vi "App -- rpr -- view optimal subspace.vi"(10 "section index":i32=9) -> (0 "Array":dbl[][](array[numeric])=[[-0.6539993268930167, 0.3391236144564683, -0.09456432043806404, 0.0051367164973633896, 0.0020044244170662685, 0.011874272381953276, 0.06955451759566218, 0.007725271948397916, -0.004046329903722955, 0.012996231366623931, 0.02336389200775809, 0.024693616597254348, -0.043124477823421006, -0.017775933941850515, 0.04206965874272625, -0.11798708971321988, -0.08203489517148861, 0.015852951226723568, -0.06159173734444465, -0.0906144627663518, -0.048921335123773224, -0.025097551631409025, 0.03747376904568885, 0.026314885922756725, -0.08142107802798851, -0.04367395508948556, 0.025063497548666342, 0.037473769045688714, -0.09061446276635161, 0.07028982367908473, -0.037287084745676984, -0.03331452126771534, -0.0014293476377641413, -0.0291901136218296, 0.0446928180029198, 0.00290562753315699, 0.012066348733460198, 0.012562461680758148, -0.018476184956469036, 0.024652499530850507, -0.00011169769376606508, -0.043673955089485336, -0.034237925342999874, -0.041796842880443226, 0.03260096402459978, 0.013337833923163239, 0.028074032981141733, 0.02479303749859956, 0.04773146565334352, -0.0917979629943126, -0.08210132900667996, 0.07469329051450514, 0.04284862090477776, -0.048649980732486074, 0.05107537884702248, -0.045809372663442795, 0.12325677070152805, 0.05609768493174689, -0.002976243880241466, 0.055086131759920394, -0.010877679296898951, -0.029218379981849323, -0.010877679296900285, -0.048682509171851414, -0.08284375332862261, 0.11159983091108487, -0.02061373332521245, 0.07830420438142319, -0.05749858935992324, 0.030209847921128213, 0.033187881765827563, 0.0632454769770712, 0.011685909194376521, 0.014141087261257316, 0.09595339373441054, 0.034766252436734583, -0.06982174337419339, -0.0082770012246038, -0.02630887225081902, -0.09198148956369846, 0.011620057966691983, 0.012656148379396237, 0.02704444806042294, -0.055089665311336876, -0.010877679296900226, 0.11265218201672413, -0.027770881489970173, 0.014843280637345453, -0.023190740122303075, 0.057998283736627604, 0.025404299712243082, 0.05096886575937984, -0.011041283301146457, -0.0785294557445813, -0.1179870897132201, 0.01825031298729252, 0.004059220722186789, 0.009722439156744988, 0.06360381321170706, -0.03557589423855971, -0.03658151530191978, -0.059497458408195626, -0.019694269436186972, 0.07525056135337402, -0.04945967745638282, 0.02704444806042326, -0.023748803061154487, 0.054380122215328834, -0.07703437213244521, 0.08566875796505154, -0.020251331993503582, -0.023952284418691773, -0.02952998594490326, 0.04206965874272611, 0.015136067978359483, -0.07102312521130782, 0.04110574188038118, -0.047734799331777364, -0.009159302165546394, 0.05123083050100717, 0.16247491505060013, -0.03658151530191925, -0.04055517231337933, -0.06397759432387508, 0.05000696501163893, -0.02274052786555141, -0.036117801828781416, 0.06438911827431076, -0.06397759432387551, 0.07902148482902957, 0.07091125409732564, 0.05660232490132762, 0.003488096034465255, 0.06098287440769287, -0.07312812028096935, -0.03997679857564285, 0.06966129911814035, -0.01200735338094387, 0.0011683041305290498, -0.026973944618607863, 0.014809638246185298, 0.05660232490132767, -0.042969630453861575, -0.0008353715209700875, -0.009143131205386776, 0.04385368363874332, 0.03122354997581172, 0.023208866857712538, -0.011927566069049402, 0.011685909194375446, 0.01752271351681508, -0.016581982918802186, 0.014945230605948495, 0.00875427084575472, 0.03168710415197408, -0.01658087713761681, -0.006730271771716752, -0.006780822682695883, -0.04222734411828173, 0.0011683041305291441, 0.04477780338783405, 0.016848841839736322, 0.024236387665468876, 0.011563814441528143, 0.08814160730020291, 0.023632730480340702, -0.019314907742346392, 0.023208866857712732, 0.01770600216283244, 0.0034828877704507445, -0.030412875700733543, 0.02234017525324682, -0.04617557628949561, -0.06294948272567681, -0.009373798802334287, 0.026878262977207832, -0.052669278619909915, -0.0038344873940750553, 0.02897704740047952, 0.0040978082744671795, 0.04452617477957913, -0.11255781245377125, 0.04010898135209824, 0.0610473165358694, 0.02223933544743438, 0.02241750520192594, -0.007179708450721197, 0.0014508139903299858, 0.02491818912257842, -0.013717635945350942, 0.02357438582599947, 0.028669025739076148, 0.0536097823579598, -0.001068008136356144, 0.038631164135670075, -0.012463770264631075, 0.01336088595160985, 0.012451807078451239, -0.03804059074580767, 0.010373724593344768, 0.025629310861148537, -0.0053638644795241846, -0.012735855163042972, -0.05318586105391781], [-0.07067784298662909, -0.07185242549664024, -0.07144584854430172, -0.07119264899191084, -0.07332609474471392, -0.07070644115676238, -0.07084424275621311, -0.07075801362519098, -0.0712278012033401, -0.07029824202490799, -0.07206471962913785, -0.07100032939852118, -0.0702926266422602, -0.07144584854430172, -0.07079246391516397, -0.07139851601076179, -0.07310747635024652, -0.07331963305869194, -0.0728467622935989, -0.07102354972586497, -0.07108171016277974, -0.07138669909159649, -0.07391572105966812, -0.06813584333743469, -0.07145769792753225, -0.07104098139347476, -0.0699417731331728, -0.07391572105966812, -0.07102354972586497, -0.07357308458233423, -0.07010256843552296, -0.07051839030505405, -0.07022535585123252, -0.0715705929812706, -0.07089037299184926, -0.07132182152419132, -0.07098293054567185, -0.0719552788008493, -0.07094238772761886, -0.07107006552052214, -0.07104679508186065, -0.07104098139347476, -0.07106424555639645, -0.07101774229969898, -0.07116339918824471, -0.07589690867298654, -0.07205253207473776, -0.07197348041419911, -0.07248324864121716, -0.07161830511784921, -0.07200385061628492, -0.07207081599015004, -0.07193103385514005, -0.07170205620150355, -0.07239641439185673, -0.07265797313696364, -0.0727773475602805, -0.07229760149533275, -0.0728657324255394, -0.07186450045604705, -0.0718886706764948, -0.07125126788349785, -0.0718886706764948, -0.07137488864390973, -0.07145177242208574, -0.07318438297654763, -0.07192497687519935, -0.07072361827988241, -0.0714399262932863, -0.07467961351717668, -0.07194315292089142, -0.07124539881911628, -0.07097713404598982, -0.07123953135154178, -0.07230376405486523, -0.0738097134634255, -0.07213187457266167, -0.07481075543571364, -0.07131004654331616, -0.07114002787526968, -0.0698150928635247, -0.07075227725677384, -0.07086153003324067, -0.07168408213995159, -0.0718886706764948, -0.07086729553974122, -0.07085576606770128, -0.07181624113087454, -0.07060936171097355, -0.07080970971931133, -0.0714340056681463, -0.07070071848804443, -0.06955851567785098, -0.07132771142643664, -0.07139851601076179, -0.07117509434956008, -0.07078671837711563, -0.07337785805054228, -0.07087883117892353, -0.07055245962799597, -0.07046172743237006, -0.07099452822109902, -0.07008031836706796, -0.07092503553925854, -0.07252679723197354, -0.07086153003324067, -0.06924603934869149, -0.0709192545777074, -0.07057520244785964, -0.07069499733747715, -0.0699086542985036, -0.06971646825442701, -0.06993072786945531, -0.07079246391516397, -0.07002479342152154, -0.07009144053179982, -0.07017504010775154, -0.07010813454135774, -0.06976572418052975, -0.0699915469448388, -0.07082696932562439, -0.07046172743237006, -0.07047304810293813, -0.07013598663994308, -0.06967823571596993, -0.06965641894431973, -0.06949349288405872, -0.06971100231169412, -0.07013598663994308, -0.06959653637490698, -0.06935327913673697, -0.06994729788712568, -0.0694017115694283, -0.06943406039089926, -0.06992520735824197, -0.06889062268192965, -0.06933178847533021, -0.069732874399712, -0.0683246384498748, -0.06848410063974669, -0.06874380846205878, -0.06994729788712568, -0.06895385031657847, -0.0696509681981926, -0.0690384432249917, -0.0693855553367308, -0.06952056189343293, -0.06818670627831608, -0.0683502785396113, -0.07097713404598982, -0.06816125981290112, -0.06852027200046291, -0.06892748293716348, -0.06768339575801093, -0.06809523917964166, -0.06912336925918049, -0.0663429299804043, -0.06828367760767108, -0.06710905713668458, -0.0683246384498748, -0.06814092423672478, -0.06639910334041323, -0.06645072443922147, -0.06837081258252144, -0.06774816568082924, -0.06748531512839379, -0.06714299243391042, -0.06818670627831608, -0.06797892627732868, -0.06705100628888166, -0.06637099837083553, -0.06515159427912529, -0.06755938232290597, -0.06754454851954433, -0.06711874748820106, -0.0682172817233295, -0.06716726466712766, -0.0677981214060557, -0.06712844219591076, -0.06614746752208296, -0.06816634670452446, -0.0700469862477013, -0.06684426460786311, -0.06985356901456403, -0.06499292371464982, -0.06696903415934995, -0.06927279934336097, -0.06700274966338278, -0.06596294552418623, -0.06483541204473581, -0.06636163818104576, -0.06625428698663569, -0.06589415478982338, -0.0669642219587416, -0.06759898908690724, -0.066582683888146, -0.06609194495907281, -0.06578910000841474, -0.06506770602475595, -0.06488778821361832, -0.06546799157784904, -0.06563020955326251, -0.06601813653815264, -0.06577543486257549]], 1 "Array of clasters":cluster{"temperature points OUT":dbl[], dbl[]}[](array[cluster])=[{"temperature points OUT"=[55.393, 55.473, 55.549, 55.623, 55.697, 55.77, 55.847, 55.926, 56.007, 56.087, 56.169, 56.251, 56.332, 56.409, 56.489, 56.565, 56.645, 56.724, 56.8, 56.877, 56.955, 57.034, 57.114, 57.191, 57.269, 57.348, 57.425, 57.505, 57.583, 57.656, 57.736, 57.815, 57.896, 57.974, 58.055, 58.137, 58.217, 58.295, 58.373, 58.45, 58.526, 58.605, 58.679, 58.759, 58.836, 58.913, 58.989, 59.071, 59.148, 59.226, 59.302, 59.381, 59.459, 59.539, 59.616, 59.694, 59.77, 59.846, 59.925, 59.998, 60.076, 60.154, 60.23, 60.308, 60.384, 60.462, 60.54, 60.618, 60.693, 60.77, 60.849, 60.928, 61.004, 61.082, 61.16, 61.239, 61.315, 61.391, 61.468, 61.544, 61.626, 61.703, 61.781, 61.86, 61.93, 62.009, 62.083, 62.162, 62.238, 62.312, 62.389, 62.466, 62.541, 62.618, 62.697, 62.774, 62.854, 63.013, 63.088, 63.165, 63.241, 63.317, 63.394, 63.472, 63.549, 63.628, 63.705, 63.782, 63.861, 63.937, 64.014, 64.089, 64.162, 64.239, 64.316, 64.393, 64.47, 64.547, 64.62, 64.696, 64.817, 64.892, 64.971, 65.046, 65.123, 65.2, 65.275, 65.35, 65.429, 65.507, 65.582, 65.655, 65.733, 65.81, 65.887, 65.965, 66.042, 66.193, 66.27, 66.345, 66.423, 66.5, 66.574, 66.651, 66.728, 66.802, 66.881, 66.956, 67.032, 67.108, 67.187, 67.258, 67.335, 67.411, 67.487, 67.563, 67.639, 67.717, 67.792, 67.869, 67.941, 68.018, 68.097, 68.174, 68.251, 68.349, 68.484, 68.558, 68.632, 68.708, 68.787, 68.864, 69.014, 69.092, 69.169, 69.246, 69.323, 69.397, 69.472, 69.546, 69.621, 69.696, 69.771, 69.845, 69.924, 69.997, 70.071, 70.149, 70.225, 70.301, 70.381, 70.457, 70.533, 70.609, 70.682, 70.76, 70.84, 70.915, 70.993, 71.145, 71.222, 71.3, 71.374, 71.452], [-1.4233131947990045, -1.44696698379756, -1.4387793210660562, -1.4336803784751888, -1.4766437933452072, -1.4238891058791603, -1.4266641599339325, -1.4249276742861876, -1.4343882750979413, -1.4156687756324693, -1.4512421714262957, -1.429807438904274, -1.4155556928348239, -1.4387793210660562, -1.4256214355869177, -1.4378261366353517, -1.472241247479028, -1.476513667656772, -1.4669909775045147, -1.430275050773841, -1.4314462879505574, -1.4375881670502726, -1.4885177113739985, -1.3721223054200284, -1.4390179444137645, -1.4306260903849541, -1.4084901910053458, -1.4885177113739985, -1.430275050773841, -1.4816176844546562, -1.411728293157671, -1.4201021303968961, -1.414200990986999, -1.4412914294668342, -1.4275931324419442, -1.4362816600343222, -1.4294570601181025, -1.449038247701824, -1.4286406072461604, -1.431211787684653, -1.43074316667139, -1.4306260903849541, -1.4310945850171213, -1.4301581005962385, -1.4330913447731966, -1.5284149458148104, -1.4509967379742121, -1.4494047925106721, -1.4596705252091262, -1.4422522583585318, -1.4500163888403113, -1.4513649401852484, -1.448550002027125, -1.4439388409904674, -1.4579218536643743, -1.4631891340084586, -1.465593100862123, -1.4559319556497243, -1.4673729987711088, -1.447210149807218, -1.447696890661646, -1.4348608480302105, -1.447696890661646, -1.4373503277880832, -1.438898616350944, -1.4737899961583356, -1.4484280263257463, -1.4242350194632807, -1.4386600585410987, -1.5039010078674286, -1.4487940562520938, -1.4347426565797863, -1.429340329978466, -1.4346244972859263, -1.4560560575170935, -1.486382926212125, -1.4525945403325102, -1.5065419490048115, -1.4360445350041873, -1.4326206923490212, -1.4059390987295817, -1.424812155072339, -1.427012291801795, -1.4435768786287146, -1.447696890661646, -1.4271283977995197, -1.4268962168360089, -1.4462383016099956, -1.4219341161639085, -1.4259687322722812, -1.438540828758084, -1.423773862550395, -1.4007721372262036, -1.436400271118469, -1.4378261366353517, -1.4333268623938835, -1.4255057317146724, -1.4776862048433326, -1.4273607029571869, -1.420788219768501, -1.4189610512278328, -1.4296906145641202, -1.4112802203999435, -1.4282911681913124, -1.4605475084505393, -1.427012291801795, -1.394479476562531, -1.428174750959171, -1.4212462155735655, -1.4236586497942072, -1.407823242604133, -1.4039529924545608, -1.4082677610481644, -1.4256214355869177, -1.4101620568525401, -1.41150419899279, -1.413187730556624, -1.411840383616908, -1.4049449102406961, -1.4094925379914167, -1.426316306906202, -1.4189610512278328, -1.4191890273390537, -1.412401270278755, -1.4031830640844094, -1.4027437170748582, -1.399462705635531, -1.4038429190838275, -1.412401270278755, -1.4015377995258496, -1.3966390756516194, -1.4086014487187513, -1.3976144098948948, -1.3982658517398951, -1.4081565887752154, -1.3873220816834984, -1.396206295863037, -1.4042833800565757, -1.3759242688543174, -1.3791355247348789, -1.384365531122584, -1.4086014487187513, -1.3885953622884066, -1.4026339497339722, -1.3902988976206005, -1.3972890550424426, -1.400007822415902, -1.3731465853332743, -1.376440609994563, -1.429340329978466, -1.3726341434072673, -1.3798639450262424, -1.3880643749598776, -1.3630108981877709, -1.3713046172859766, -1.392009141452825, -1.3360165453917334, -1.3750993977955097, -1.3514448443373293, -1.3759242688543174, -1.372224624770697, -1.3371477667352039, -1.3381873144627388, -1.3768541253620603, -1.3643152374527774, -1.3590219426416679, -1.3521282346937675, -1.3731465853332743, -1.3689623034632596, -1.3502758140704776, -1.3365817877473203, -1.3120253799654444, -1.360513510731414, -1.3602147870131798, -1.3516399890190685, -1.3737623148530995, -1.3526170298853801, -1.3653212478213177, -1.351835221425999, -1.3320803146826385, -1.372736583431779, -1.410608976863067, -1.3461124419290225, -1.4067139329795428, -1.308830065868396, -1.3486250560869568, -1.3950183703925685, -1.3493040202393891, -1.3283644033978703, -1.3056580896358188, -1.3363932918754797, -1.3342314492806202, -1.3269790928711038, -1.3485281478009576, -1.3613111133098765, -1.3408447190593702, -1.3309621991148441, -1.324863495532006, -1.3103360349842297, -1.3067128429943444, -1.3183970012691315, -1.32166375326782, -1.32947584221792, -1.3245883062851367]}], 11 "9w folder path":path=path "E:/data/Ultrasound/Experiment/ProbeTest/Probe10/YBCO_5/sweep5/9w")   [LabVIEW 2014]
uses:
  link -- rusout - tetragonal.ctl
  cursor winow.ctl
  query.ctl
  cursor window action.ctl
  <vilib>/Analysis/baseanly.llb/Real A x B.vi
  <vilib>/Utility/file.llb/Write To Spreadsheet File (DBL).vi
  <vilib>/Analysis/Matrix/Numeric/Conversions/Array To Matrix - RA2.vi
  <vilib>/Analysis/Matrix/Numeric/Conversions/Matrix To Array - RM.vi
  <vilib>/Analysis/Matrix/NI_Matrix.lvlib
  <vilib>/Analysis/NI_AALBase.lvlib
panel:
  in  "Tab Control 2":enum32{"Page 1", "Page 2"}(tab)
  out "Plot:   what vs temp 2":cluster{dbl[], dbl[]}[](graph)=[{[60.693, 60.77, 60.849, 60.928, 61.004, 61.082, 61.16, 61.239, 61.315, 61.391, 61.468, 61.544, 61.626, 61.703, 61.781, 61.86, 61.93, 62.009, 62.083, 62.162, 62.238, 62.312, 62.389, 62.466, 62.541, 62.618, 62.697, 62.774, 62.854, 62.932, 63.013, 63.088, 63.165, 63.241, 63.317, 63.394, 63.472, 63.549], [-0.0004933279279327732, -0.0004959461002016808, -0.0004987375917983193, -0.0005013767724705882, -0.0005039476758319328, -0.0005070674237310925, -0.0005096724657478992, -0.0005120936842352941, -0.0005132649027226891, -0.0005130075497815126, -0.0005117076548235294, -0.0005095096506218488, -0.0005068126968403361, -0.0005043625917983194, -0.0005024770875966387, -0.0005009854909579832, -0.0005000269825546219, -0.0004992365413781513, -0.0004986719405378152, -0.0004978683691092438, -0.0004972249867563025, -0.000496810070789916, -0.0004963557640672269, -0.000495951352302521, -0.0004956414783529412, -0.0004949140623865546, -0.0004947512472605043, -0.0004943310791932774, -0.0004938058691092437, -0.0004934907430588235, -0.000493107339697479, -0.0004928132220504202, -0.0004925007220504202, -0.0004922880119663866, -0.0004920805539831933, -0.0004917207850756302, -0.0004911640623865547, -0.000490856814487395]}, {[60.693, 60.77, 60.849, 60.928, 61.004, 61.082, 61.16], [-0.0004933414395167107, -0.0004959475211230401, -0.0004986595074246494, -0.0005014110372937718, -0.0005040962098828075, -0.0005068917751889707, -0.0005097284672831535]}, {[61.391, 61.468, 61.544, 61.626, 61.703, 61.781], [-0.0005134949407613455, -0.0005112990207351107, -0.00050914039550645, -0.0005068210704880685, -0.0005046522940388857, -0.0005024643077469364]}]
  out "best fit parameters right":dbl[](array[numeric])=[0.000561899976493353, -0.040468997251097254, -37.63175425304014]
  out "best fit parameters left":dbl[](array[numeric])=[-0.0001212473626486651, -0.0041194510604749875, -10.603993376591303]
  in  "gap":dbl=1.0
  out "residue right":dbl=1.0417365940205689e-13
  out "residue left":dbl=9.072396572402669e-15
  out "x-y":dbl[](array[numeric])=[-3.1383182947303852e-06, -3.7664734781920825e-06, 1.2053722232650138e-06]
  out "Plot:   LandauKhalat":cluster{"Array":dbl[], dbl[]}[](graph)
  out "Plot:   optimal subspace derivative":cluster{dbl[], dbl[]}[](graph)=[{[55.393, 55.473, 55.549, 55.623, 55.697, 55.77, 55.847, 55.926, 56.007, 56.087, 56.169, 56.251, 56.332, 56.409, 56.489, 56.565, 56.645, 56.724, 56.8, 56.877, 56.955, 57.034, 57.114, 57.191, 57.269, 57.348, 57.425, 57.505, 57.583, 57.656, 57.736, 57.815, 57.896, 57.974, 58.055, 58.137, 58.217, 58.295, 58.373, 58.45, 58.526, 58.605, 58.679, 58.759, 58.836, 58.913, 58.989, 59.071, 59.148, 59.226, 59.302, 59.381, 59.459, 59.539, 59.616, 59.694, 59.77, 59.846, 59.925, 59.998, 60.076, 60.154, 60.23, 60.308, 60.384, 60.462, 60.54, 60.618, 60.693, 60.77, 60.849, 60.928, 61.004, 61.082, 61.16, 61.239, 61.315, 61.391, 61.468, 61.544, 61.626, 61.703, 61.781, 61.86, 61.93, 62.009, 62.083, 62.162, 62.238, 62.312, 62.389, 62.466, 62.541, 62.618, 62.697, 62.774, 62.854, 63.013, 63.088, 63.165, 63.241, 63.317, 63.394, 63.472, 63.549, 63.628, 63.705, 63.782, 63.861, 63.937, 64.014, 64.089, 64.162, 64.239, 64.316, 64.393, 64.47, 64.547, 64.62, 64.696, 64.817, 64.892, 64.971, 65.046, 65.123, 65.2, 65.275, 65.35, 65.429, 65.507, 65.582, 65.655, 65.733, 65.81, 65.887, 65.965, 66.042, 66.193, 66.27, 66.345, 66.423, 66.5, 66.574, 66.651, 66.728, 66.802, 66.881, 66.956, 67.032, 67.108, 67.187, 67.258, 67.335, 67.411, 67.487, 67.563, 67.639, 67.717, 67.792, 67.869, 67.941, 68.018, 68.097, 68.174, 68.251, 68.349, 68.484, 68.558, 68.632, 68.708, 68.787, 68.864, 69.014, 69.092, 69.169, 69.246, 69.323, 69.397, 69.472, 69.546, 69.621, 69.696, 69.771, 69.845, 69.924, 69.997, 70.071, 70.149, 70.225, 70.301, 70.381, 70.457, 70.533, 70.609, 70.682, 70.76, 70.84, 70.915, 70.993, 71.145, 71.222, 71.3, 71.374, 71.452], [0.0, 12.414036766868827, -5.706420195980651, 1.3473113099382437, -0.04232827135536354, 0.13520339677927334, 0.7490940936845489, -0.7826486790792884, -0.1453284179274254, 0.21303201587932172, 0.12643488586749957, 0.016216153530442028, -0.8372604249465776, 0.3292018685918323, 0.7480699085572255, -2.10600984810454, 0.4494024317716105, 1.2390866632686104, -1.0190090601469433, -0.3769185119727942, 0.5345272774689844, 0.30156687965017737, 0.7821415084637401, -0.14492056003806963, -1.3812303070609098, 0.47781168276585634, 0.8926941901058899, 0.15512839371276918, -1.6421568181031685, 2.204168307471719, -1.3447113553095502, 0.05028561364508367, 0.3936441188882715, -0.35590725620598634, 0.912134958330205, -0.5095998837775906, 0.11450901500379254, 0.00636042240125553, -0.39793136714395944, 0.560112785549566, -0.3258447003239001, -0.5514209796926942, 0.12751391549303787, -0.09448646921804392, 0.9662052844811007, -0.250170520797883, 0.1938973560260315, -0.04001214003100173, 0.2979016643473037, -1.7888388288161992, 0.12758728931095492, 1.984742019255492, -0.4082649949964895, -1.1437325204658224, 1.2951345399936482, -1.2421121988520718, 2.2245545179601276, -0.8836721811814078, -0.7477712507846568, 0.7953750087693362, -0.8456898853438056, -0.2351371882685856, 0.24132500901250825, -0.4846773060890987, -0.44949005469435477, 2.4928664646115397, -1.6950456953372353, 1.2681786885465627, -1.8107039165513887, 1.1390706140395512, 0.03769663094556448, 0.3804758887499164, -0.6784153655617674, 0.031476641883085923, 1.0488757240148407, -0.7745207759199427, -1.376157839617464, 0.8097992388103838, -0.23418014319758418, -0.8641133856958572, 1.2634335064681648, 0.013455719645508873, 0.18446538052599318, -1.0396723211615084, 0.6315998002062353, 1.5636691305521946, -1.8976089663067295, 0.5394197737634847, -0.5004476415743193, 1.0971489710666593, -0.42329849382314655, 0.33200735126152414, -0.8268019874737309, -0.8764697719926001, -0.49946372112200615, 1.7693169181885176, -0.17738865331382542, 0.03561772600351092, 0.7184183207328004, -1.2880481487047937, -0.013231856096842968, -0.301525567187838, 0.5169245321040208, 1.217241420378941, -1.6196134910358415, 0.9684066521114617, -0.6596526119685577, 1.0146613672270801, -1.6634746119971267, 2.1408306591775745, -1.3755855838773716, -0.04934603233584067, -0.07640687022206732, 0.92986551542378, -0.34978689304373073, -1.1189505609047967, 1.4562190531388528, -1.1537732624955928, 0.528431468030507, 0.7946070087705105, 0.9193725995834501, -2.654085738033491, -0.05029945584126193, -0.31229896013993147, 1.4803189524093079, -0.9447726347687281, -0.17836365284306002, 1.3400922680414322, -1.624895096179414, 1.8333215276012778, -0.10813640975606878, -0.1960127287122815, -0.6809516521392353, 0.7466854334185582, -1.741701229722927, 0.42501694494006725, 1.4238713986205946, -0.540852003305207, 0.17111243521393807, -0.3752299833218113, 0.5356869598050202, 0.5427621643525111, -1.3455669642593493, 0.5471981679596426, -0.10789298291450498, 0.7161731735692067, -0.15987510965737514, -0.1068624415746517, -0.4623214858784867, 0.3107036218871379, 0.07388359901822927, -0.48034783712138385, 0.4094443314902782, -0.08145999684464678, 0.30174780666080725, -0.6351050169682376, 0.12961322849869622, -0.0006480886022965323, -0.47262028580779336, 0.5635798473871676, 0.6056874896847674, -0.3627137863389401, 0.09351323830041974, -0.16457887303816485, 0.9945167903724231, -0.6582538451006417, -0.3181306535014073, 0.5746456027034064, -0.07436303641730319, -0.18714624200503854, -0.4290602971035566, 0.685104557843917, -0.45677167695164217, -0.21505008251513544, 0.6957881029005687, 0.4708059971369218, -1.0330849558067483, 0.6599296111598211, 0.43748713059412736, -0.33620593413524613, 0.5390448867349077, -2.094453163111259, 2.0355572507448496, 0.2829504754563744, -0.4912402669421674, 0.002440681568377736, -0.39996234665740416, 0.1106477236032161, 0.30878125174013776, -0.5083661193148091, 0.46615027214189003, 0.06703473569838315, 0.32816785024843625, -0.7194446117673775, 0.5438242776989334, -0.6550632615422975, 0.3228082027030184, -0.012121051642114345, -0.6473384336444384, 0.3185152324944218, 0.1981244969844692, -0.39734840180348135, -0.09962149572322947, -0.5185898191137603]}, ...(2 in all)]
  out "standard error":string
  out "standard output":string
  out "string":string
  out "name":string
  out "Numeric":i32=1
  out "common  freq points":dbl[][](array[numeric])=[[-1.4233131947990045, -1.44696698379756, -1.4387793210660562, -1.4336803784751888, -1.4766437933452072, -1.4238891058791603, -1.4266641599339325, -1.4249276742861876, -1.4343882750979413, -1.4156687756324693, -1.4512421714262957, -1.429807438904274, -1.4155556928348239, -1.4387793210660562, -1.4256214355869177, -1.4378261366353517, -1.472241247479028, -1.476513667656772, -1.4669909775045147, -1.430275050773841, -1.4314462879505574, -1.4375881670502726, -1.4885177113739985, -1.3721223054200284, -1.4390179444137645, -1.4306260903849541, -1.4084901910053458, -1.4885177113739985, -1.430275050773841, -1.4816176844546562, -1.411728293157671, -1.4201021303968961, -1.414200990986999, -1.4412914294668342, -1.4275931324419442, -1.4362816600343222, -1.4294570601181025, -1.449038247701824, -1.4286406072461604, -1.431211787684653, -1.43074316667139, -1.4306260903849541, -1.4310945850171213, -1.4301581005962385, -1.4330913447731966, -1.5284149458148104, -1.4509967379742121, -1.4494047925106721, -1.4596705252091262, -1.4422522583585318, -1.4500163888403113, -1.4513649401852484, -1.448550002027125, -1.4439388409904674, -1.4579218536643743, -1.4631891340084586, -1.465593100862123, -1.4559319556497243, -1.4673729987711088, -1.447210149807218, -1.447696890661646, -1.4348608480302105, -1.447696890661646, -1.4373503277880832, -1.438898616350944, -1.4737899961583356, -1.4484280263257463, -1.4242350194632807, -1.4386600585410987, -1.5039010078674286, -1.4487940562520938, -1.4347426565797863, -1.429340329978466, -1.4346244972859263, -1.4560560575170935, -1.486382926212125, -1.4525945403325102, -1.5065419490048115, -1.4360445350041873, -1.4326206923490212, -1.4059390987295817, -1.424812155072339, -1.427012291801795, -1.4435768786287146, -1.447696890661646, -1.4271283977995197, -1.4268962168360089, -1.4462383016099956, -1.4219341161639085, -1.4259687322722812, -1.438540828758084, -1.423773862550395, -1.4007721372262036, -1.436400271118469, -1.4378261366353517, -1.4333268623938835, -1.4255057317146724, -1.4776862048433326, -1.4273607029571869, -1.420788219768501, -1.4189610512278328, -1.4296906145641202, -1.4112802203999435, -1.4282911681913124, -1.4605475084505393, -1.427012291801795, -1.394479476562531, -1.428174750959171, -1.4212462155735655, -1.4236586497942072, -1.407823242604133, -1.4039529924545608, -1.4082677610481644, -1.4256214355869177, -1.4101620568525401, -1.41150419899279, -1.413187730556624, -1.411840383616908, -1.4049449102406961, -1.4094925379914167, -1.426316306906202, -1.4189610512278328, -1.4191890273390537, -1.412401270278755, -1.4031830640844094, -1.4027437170748582, -1.399462705635531, -1.4038429190838275, -1.412401270278755, -1.4015377995258496, -1.3966390756516194, -1.4086014487187513, -1.3976144098948948, -1.3982658517398951, -1.4081565887752154, -1.3873220816834984, -1.396206295863037, -1.4042833800565757, -1.3759242688543174, -1.3791355247348789, -1.384365531122584, -1.4086014487187513, -1.3885953622884066, -1.4026339497339722, -1.3902988976206005, -1.3972890550424426, -1.400007822415902, -1.3731465853332743, -1.376440609994563, -1.429340329978466, -1.3726341434072673, -1.3798639450262424, -1.3880643749598776, -1.3630108981877709, -1.3713046172859766, -1.392009141452825, -1.3360165453917334, -1.3750993977955097, -1.3514448443373293, -1.3759242688543174, -1.372224624770697, -1.3371477667352039, -1.3381873144627388, -1.3768541253620603, -1.3643152374527774, -1.3590219426416679, -1.3521282346937675, -1.3731465853332743, -1.3689623034632596, -1.3502758140704776, -1.3365817877473203, -1.3120253799654444, -1.360513510731414, -1.3602147870131798, -1.3516399890190685, -1.3737623148530995, -1.3526170298853801, -1.3653212478213177, -1.351835221425999, -1.3320803146826385, -1.372736583431779, -1.410608976863067, -1.3461124419290225, -1.4067139329795428, -1.308830065868396, -1.3486250560869568, -1.3950183703925685, -1.3493040202393891, -1.3283644033978703, -1.3056580896358188, -1.3363932918754797, -1.3342314492806202, -1.3269790928711038, -1.3485281478009576, -1.3613111133098765, -1.3408447190593702, -1.3309621991148441, -1.324863495532006, -1.3103360349842297, -1.3067128429943444, -1.3183970012691315, -1.32166375326782, -1.32947584221792, -1.3245883062851367]]
  in  "Tab Control":T1(tab)
  in  "temperature mapping":bool
  in  "dump optimal vectors":bool
  in  "misc controls":T2[](array[typedef])=[{"Boolean"=FALSE, "String"="calc el consts"}, {"Boolean"=FALSE, "String"="read rusout file"}, {"Boolean"=FALSE, "String"="export plot "}, {"Boolean"=FALSE, "String"="critical"}]
  in  "buttons 4":bool[](array[boolean])=[FALSE, FALSE, TRUE, TRUE, TRUE, FALSE, FALSE, TRUE, FALSE, FALSE, TRUE, TRUE, FALSE, FALSE, FALSE, TRUE]
  in  "active":bool[](array[boolean])=[FALSE, TRUE, FALSE, FALSE]
  in  "buttons 3":bool[](array[boolean])=[FALSE, FALSE, FALSE, TRUE, FALSE, FALSE, FALSE, FALSE, FALSE, FALSE, FALSE, FALSE, FALSE, FALSE, FALSE, FALSE, FALSE, FALSE, FALSE, FALSE, FALSE, FALSE]
  in  "buttons 2":bool[](array[boolean])=[TRUE, TRUE, TRUE, TRUE, TRUE, TRUE, FALSE, TRUE, TRUE, FALSE, TRUE, TRUE, TRUE, TRUE, TRUE, TRUE, TRUE, TRUE, FALSE, FALSE, FALSE, FALSE]
  in  "show plot pallettes":bool
  out "Plot:   what vs temp":cluster{dbl[], dbl[]}[](graph)=[{[55.393, 55.473, 55.549, 55.623, 55.697, 55.77, 55.847, 55.926, 56.007, 56.087, 56.169, 56.251, 56.332, 56.409, 56.489, 56.565, 56.645, 56.724, 56.8, 56.877, 56.955, 57.034, 57.114, 57.191, 57.269, 57.348, 57.425, 57.505, 57.583, 57.656, 57.736, 57.815, 57.896, 57.974, 58.055, 58.137, 58.217, 58.295, 58.373, 58.45, 58.526, 58.605, 58.679, 58.759, 58.836, 58.913, 58.989, 59.071, 59.148, 59.226, 59.302, 59.381, 59.459, 59.539, 59.616, 59.694, 59.77, 59.846, 59.925, 59.998, 60.076, 60.154, 60.23, 60.308, 60.384, 60.462, 60.54, 60.618, 60.693, 60.77, 60.849, 60.928, 61.004, 61.082, 61.16, 61.239, 61.315, 61.391, 61.468, 61.544, 61.626, 61.703, 61.781, 61.86, 61.93, 62.009, 62.083, 62.162, 62.238, 62.312, 62.389, 62.466, 62.541, 62.618, 62.697, 62.774, 62.854, 63.013, 63.088, 63.165, 63.241, 63.317, 63.394, 63.472, 63.549, 63.628, 63.705, 63.782, 63.861, 63.937, 64.014, 64.089, 64.162, 64.239, 64.316, 64.393, 64.47, 64.547, 64.62, 64.696, 64.817, 64.892, 64.971, 65.046, 65.123, 65.2, 65.275, 65.35, 65.429, 65.507, 65.582, 65.655, 65.733, 65.81, 65.887, 65.965, 66.042, 66.193, 66.27, 66.345, 66.423, 66.5, 66.574, 66.651, 66.728, 66.802, 66.881, 66.956, 67.032, 67.108, 67.187, 67.258, 67.335, 67.411, 67.487, 67.563, 67.639, 67.717, 67.792, 67.869, 67.941, 68.018, 68.097, 68.174, 68.251, 68.349, 68.484, 68.558, 68.632, 68.708, 68.787, 68.864, 69.014, 69.092, 69.169, 69.246, 69.323, 69.397, 69.472, 69.546, 69.621, 69.696, 69.771, 69.845, 69.924, 69.997, 70.071, 70.149, 70.225, 70.301, 70.381, 70.457, 70.533, 70.609, 70.682, 70.76, 70.84, 70.915, 70.993, 71.145, 71.222, 71.3, 71.374, 71.452], [-1.4233131928950045, -1.44696698189356, -1.4387793191620561, -1.4336803765711887, -1.4766437914412072, -1.4238891039751602, -1.4266641580299324, -1.4249276723821875, -1.4343882731939412, -1.4156687737284692, -1.4512421695222957, -1.429807437000274, -1.4155556909308238, -1.4387793191620561, -1.4256214336829176, -1.4378261347313517, -1.472241245575028, -1.476513665752772, -1.4669909756005146, -1.430275048869841, -1.4314462860465573, -1.4375881651462725, -1.4885177094699984, -1.3721223035160284, -1.4390179425097644, -1.430626088480954, -1.4084901891013457, -1.4885177094699984, -1.430275048869841, -1.4816176825506562, -1.4117282912536708, -1.420102128492896, -1.414200989082999, -1.4412914275628341, -1.4275931305379441, -1.4362816581303222, -1.4294570582141024, -1.449038245797824, -1.4286406053421603, -1.431211785780653, -1.4307431647673898, -1.430626088480954, -1.4310945831131212, -1.4301580986922384, -1.4330913428691965, -1.5284149439108103, -1.450996736070212, -1.449404790606672, -1.4596705233051261, -1.4422522564545317, -1.4500163869363112, -1.4513649382812484, -1.4485500001231248, -1.4439388390864674, -1.4579218517603743, -1.4631891321044586, -1.465593098958123, -1.4559319537457243, -1.4673729968671088, -1.447210147903218, -1.447696888757646, -1.4348608461262105, -1.447696888757646, -1.4373503258840832, -1.438898614446944, -1.4737899942543355, -1.4484280244217462, -1.4242350175592806, -1.4386600566370986, -1.5039010059634286, -1.4487940543480937, -1.4347426546757862, -1.4293403280744659, -1.4346244953819263, -1.4560560556130935, -1.486382924308125, -1.4525945384285102, -1.5065419471008115, -1.4360445331001872, -1.4326206904450212, -1.4059390968255816, -1.4248121531683389, -1.4270122898977948, -1.4435768767247146, -1.447696888757646, -1.4271283958955197, -1.4268962149320088, -1.4462382997059955, -1.4219341142599085, -1.425968730368281, -1.438540826854084, -1.423773860646395, -1.4007721353222036, -1.4364002692144688, -1.4378261347313517, -1.4333268604898834, -1.4255057298106724, -1.4776862029393325, -1.4273607010531868, -1.4207882178645008, -1.4189610493238327, -1.42969061266012, -1.4112802184959434, -1.4282911662873123, -1.4605475065465392, -1.4270122898977948, -1.394479474658531, -1.4281747490551708, -1.4212462136695654, -1.4236586478902071, -1.407823240700133, -1.4039529905505608, -1.4082677591441644, -1.4256214336829176, -1.41016205494854, -1.4115041970887898, -1.413187728652624, -1.411840381712908, -1.404944908336696, -1.4094925360874166, -1.4263163050022019, -1.4189610493238327, -1.4191890254350537, -1.4124012683747549, -1.4031830621804093, -1.4027437151708582, -1.399462703731531, -1.4038429171798275, -1.4124012683747549, -1.4015377976218495, -1.3966390737476193, -1.4086014468147512, -1.3976144079908948, -1.398265849835895, -1.4081565868712154, -1.3873220797794983, -1.396206293959037, -1.4042833781525756, -1.3759242669503173, -1.3791355228308788, -1.384365529218584, -1.4086014468147512, -1.3885953603844066, -1.402633947829972, -1.3902988957166005, -1.3972890531384425, -1.400007820511902, -1.3731465834292742, -1.376440608090563, -1.4293403280744659, -1.3726341415032672, -1.3798639431222424, -1.3880643730558775, -1.3630108962837708, -1.3713046153819766, -1.392009139548825, -1.3360165434877334, -1.3750993958915096, -1.3514448424333292, -1.3759242669503173, -1.372224622866697, -1.3371477648312038, -1.3381873125587387, -1.3768541234580602, -1.3643152355487773, -1.3590219407376678, -1.3521282327897675, -1.3731465834292742, -1.3689623015592596, -1.3502758121664775, -1.3365817858433202, -1.3120253780614444, -1.3605135088274138, -1.3602147851091797, -1.3516399871150684, -1.3737623129490995, -1.35261702798138, -1.3653212459173176, -1.351835219521999, -1.3320803127786385, -1.372736581527779, -1.410608974959067, -1.3461124400250224, -1.4067139310755428, -1.308830063964396, -1.3486250541829568, -1.3950183684885684, -1.349304018335389, -1.3283644014938703, -1.3056580877318187, -1.3363932899714797, -1.3342314473766201, -1.3269790909671038, -1.3485281458969576, -1.3613111114058765, -1.3408447171553701, -1.330962197210844, -1.324863493628006, -1.3103360330802296, -1.3067128410903444, -1.3183969993651314, -1.3216637513638199, -1.32947584031392, -1.3245883043811366]}]
  in  "buttons 1":bool[](array[boolean])=[TRUE, TRUE, TRUE, TRUE, TRUE, TRUE, TRUE, TRUE, TRUE, FALSE, TRUE, TRUE, TRUE, TRUE, TRUE, TRUE, TRUE, FALSE, FALSE, FALSE, TRUE, TRUE]
  out "all peaks":i32[](array[numeric])=[1589, 1766, 1825, 1904, 2037, 2462, 2972, 3131]
  out "all peaks exp":i32[](array[numeric])=[564, 649, 987, 1133, 1214, 1585, 1763, 1823, 1880, 1899, 2032, 2138, 2221, 2270, 2350, 2456, 2580, 2634, 2831, 2960, 2965, 3131, 3328, 3469, 3553, 0, 3615, 3734, 0, 0, 0, 4236, 4300, 4331]
  out "Plot:   what vs temp (all points)":cluster{dbl[], dbl[]}[](graph)
  out "Plot:   elastic vs temp":cluster{dbl[], dbl[]}[](graph)=[{[46.762, 47.022, 47.27, 47.517, 47.768, 48.03, 48.278, 48.522, 48.777, 49.026, 49.27, 49.522, 49.772, 50.025, 50.288, 50.534, 50.8, 51.05, 51.303, 51.563, 51.816, 52.08, 52.341, 52.605, 52.863, 53.113, 53.366, 53.624, 53.877, 54.135, 54.389, 54.652, 54.907, 55.16, 55.425, 55.68, 55.936, 56.19, 56.46, 56.719, 56.975, 57.228, 57.492, 57.746, 58.001, 58.265, 58.52, 58.774, 59.032, 59.296, 59.551, 59.801, 60.051, 60.311, 60.562, 60.813, 61.064, 61.32, 61.568, 61.816, 62.07, 62.319, 62.573, 62.819, 63.082, 63.334, 63.583, 63.836, 64.094, 64.347, 64.593, 64.857, 65.106, 65.358, 65.61, 65.87, 66.118, 66.367, 66.614, 66.87, 67.115, 67.36, 67.606, 67.859, 68.106, 68.352, 68.611, 68.86, 69.107, 69.355, 69.61, 69.857, 70.103, 70.35, 70.606, 70.853, 71.098, 71.348, 71.605, 71.853, 72.102, 72.356, 72.599, 72.844, 73.085, 73.338, 73.581, 73.825, 74.071, 74.329, 74.572, 74.815, 75.068, 75.315, 75.558, 75.803, 76.056, 76.3, 76.545, 76.787, 77.041, 77.284, 77.53, 77.779, 78.034, 78.279, 78.524, 78.778, 79.023, 79.265, 79.507, 79.759, 80.003, 80.245, 80.484, 80.741, 80.981, 81.226, 81.481, 81.722, 81.962, 82.202, 82.45, 82.69, 82.928, 83.167, 83.417, 83.662, 83.903, 84.147, 84.401, 84.644, 84.887, 85.141, 85.389, 85.635, 85.884, 86.14, 86.39], [-0.004996303090462477, -0.004974409084222285, -0.004977647809396878, -0.004951528092668833, -0.004948078941049739, -0.004924059659124823, -0.0049103650924231385, -0.0049007463930566654, -0.004892649984805305, -0.004882898874673165, -0.004865120969543957, -0.004858001116073973, -0.004834064614128542, -0.004837530354647013, -0.0048096803225681755, -0.004800750425676709, -0.004798418070929126, -0.004798378007124668, -0.004771341847788444, -0.004755367332219322, -0.004738471818122211, -0.004740332198340772, -0.004714803063477505, -0.004705425271209356, -0.004702506539017068, -0.004678516733746472, -0.0046681861160614456, -0.004627545305465525, -0.004633243153386733, -0.004610618671944745, -0.0045614917539248175, -0.00459371042817849, -0.004621312699181377, -0.004540598294661305, -0.004582671731702722, -0.004577146232960891, -0.004528214954210549, -0.00460645967315661, -0.004561975497599929, -0.0045524636185688755, -0.004552063748413697, -0.004544451428787935, -0.004591158479345356, -0.004596828551209256, -0.004550333402205631, -0.004589225311561197, -0.004523648635915763, -0.004609015071072343, -0.004606579355138346, -0.0045710541234597795, -0.004609753303391261, -0.004608341986305222, -0.004612274593658225, -0.004613509657026953, -0.004618338629921643, -0.004609427450992914, -0.004606780991939365, -0.004600351717957624, -0.0045959493272975166, -0.004565441847418316, -0.004563488524663832, -0.00461246723718449, -0.004607887922699873, -0.004618560286871433, -0.00456359846325418, -0.004598063296514359, -0.004572417638416007, -0.004608710281392586, -0.004570171821602829, -0.00461137263597104, -0.00460613011735971, -0.004599925668532278, -0.004590576498554796, -0.004587090225983346, -0.004589288557582328, -0.004596129828901566, -0.0046074351606803406, -0.0045758919061712625, -0.004572845159556083, -0.0046011630143717565, -0.004607859313982496, -0.004617906019421444, -0.004576251650243583, -0.004610705624463876, -0.004602234445501804, -0.004621876548378838, -0.004622045991871526, -0.00458462886293759, -0.0045818021961706356, -0.0045878844980277575, -0.004591381053544575, -0.004596062264433549, -0.004603204927664598, -0.004594006095569566, -0.004585851876270199, -0.004653372459320538, -0.004622993220393298, -0.004639063008900034, -0.004653470822853062, -0.004662844367993445, -0.00466876479498491, -0.004685860166262993, -0.004704617586663742, -0.004694382488932131, -0.004700239906425937, -0.004705347877124738, -0.004697105311847469, -0.00469517652643764, -0.0046862605629710025, -0.004688712061492811, -0.004692175859485092, -0.004701454991976498, -0.004709266499505082, -0.004695103765708046, -0.004692477099507669, -0.004711207956905415, -0.00469977147064731, -0.0047153840845944655, -0.004728622689274412, -0.004731423424832434, -0.0047442008098061384, -0.004750513689825545, -0.004767560344673281, -0.004777897801055176, -0.004776068703649752, -0.004789024643916694, -0.004792903118296445, -0.004819457209393847, -0.0048365771171231114, -0.0048400787636397125, -0.004850122544471912, -0.004870738905257208, -0.0048639261349874485, -0.004882494972807557, -0.004899235474529698, -0.004903380845833091, -0.004909259730730224, -0.004911103181313558, -0.004928273840377569, -0.004933652472439714, -0.004933201083384766, -0.004955398329006135, -0.004966122050717865, -0.004964743871664117, -0.0049879386755120134, -0.00499234869419784, -0.004998790929563304, -0.005022634039460745, -0.005037781429465679, -0.005045148462827321, -0.005053026444809165, -0.005074862965547495, -0.005087981561601077, -0.005101798600012244, -0.005130650723619712, -0.005135866035161232, -0.005163538031184386, -0.005181044665526532, -0.005199765059712416]}, {[46.762, 47.022, 47.27, 47.517, 47.768, 48.03, 48.278, 48.522, 48.777, 49.026, 49.27, 49.522, 49.772, 50.025, 50.288, 50.534, 50.8, 51.05, 51.303, 51.563, 51.816, 52.08, 52.341, 52.605, 52.863, 53.113, 53.366, 53.624, 53.877, 54.135, 54.389, 54.652, 54.907, 55.16, 55.425, 55.68, 55.936, 56.19, 56.46, 56.719, 56.975, 57.228, 57.492, 57.746, 58.001, 58.265, 58.52, 58.774, 59.032, 59.296, 59.551, 59.801, 60.051, 60.311, 60.562, 60.813, 61.064, 61.32, 61.568, 61.816, 62.07, 62.319, 62.573, 62.819, 63.082, 63.334, 63.583, 63.836, 64.094, 64.347, 64.593, 64.857, 65.106, 65.358, 65.61, 65.87, 66.118, 66.367, 66.614, 66.87, 67.115, 67.36, 67.606, 67.859, 68.106, 68.352, 68.611, 68.86, 69.107, 69.355, 69.61, 69.857, 70.103, 70.35, 70.606, 70.853, 71.098, 71.348, 71.605, 71.853, 72.102, 72.356, 72.599, 72.844, 73.085, 73.338, 73.581, 73.825, 74.071, 74.329, 74.572, 74.815, 75.068, 75.315, 75.558, 75.803, 76.056, 76.3, 76.545, 76.787, 77.041, 77.284, 77.53, 77.779, 78.034, 78.279, 78.524, 78.778, 79.023, 79.265, 79.507, 79.759, 80.003, 80.245, 80.484, 80.741, 80.981, 81.226, 81.481, 81.722, 81.962, 82.202, 82.45, 82.69, 82.928, 83.167, 83.417, 83.662, 83.903, 84.147, 84.401, 84.644, 84.887, 85.141, 85.389, 85.635, 85.884, 86.14, 86.39], [-0.0074751179184890165, -0.007454869960650559, -0.007439610824147112, -0.007396558451555666, -0.0073789244292177735, -0.007348143738536286, -0.007319503775637461, -0.007305285419676557, -0.007289623659700728, -0.007268053667391339, -0.007236518623091589, -0.007224640267161047, -0.007184548049735562, -0.007185222013659226, -0.007142548741229405, -0.007128616299502868, -0.007125590847323483, -0.007114273596882043, -0.007086361317137906, -0.007055313898910002, -0.00702805546543021, -0.007026718911975553, -0.006991487761406531, -0.006965342705076881, -0.00696368089658803, -0.006924427752241711, -0.006906637722927695, -0.006843352479839117, -0.006850298599848982, -0.006816574123554275, -0.006743862490085155, -0.006787254989797025, -0.0068177798181043745, -0.006687257868531971, -0.006750053339056411, -0.006730206359478056, -0.006655629260399067, -0.00675054546396912, -0.0066724269289965875, -0.00664989909967299, -0.006636406361804827, -0.0066140319975444475, -0.00666247975217907, -0.006650466916034261, -0.006572203257657066, -0.006610839123848574, -0.0065012946516904355, -0.006597632612592973, -0.006578938856593465, -0.006511522186596842, -0.006546737237986009, -0.006529637786821966, -0.006510679178634685, -0.006492540701970545, -0.006475767169281022, -0.006446736850017134, -0.006414091278315658, -0.006388945609486166, -0.006391462190708501, -0.006358120029477624, -0.006359559869108767, -0.006427354314173723, -0.00642533827219751, -0.006435660759398941, -0.006366147559359873, -0.0064173107344916575, -0.006377758340634211, -0.006421656059586374, -0.006373497121998677, -0.006428651610219352, -0.006425479433025875, -0.006422170517895276, -0.006413042556950738, -0.006408598043322547, -0.006416351832580598, -0.006426939708948651, -0.006440926741929173, -0.006390392853638044, -0.0063848684648669446, -0.006429155543506635, -0.006439713947488001, -0.006451617324579379, -0.006397330642446014, -0.006446646535028174, -0.006438612627960853, -0.006457384314170279, -0.0064642111722097795, -0.006412009989637731, -0.006412320110703514, -0.006419436920679206, -0.006430199347309368, -0.006432503907292673, -0.006438815186566714, -0.006432167523982745, -0.00642393920288778, -0.00650934984025185, -0.006468188466920076, -0.006489011745804127, -0.006506809150184949, -0.006515900111928637, -0.0065222199552878845, -0.006543064215880634, -0.006564879955868446, -0.006554342150281646, -0.0065624875763314475, -0.0065737323211392164, -0.006566696023794306, -0.006572174521946263, -0.006558438500873762, -0.0065650100926328316, -0.006574822052096891, -0.006588236948224809, -0.006601810519031722, -0.006589457665750228, -0.006587676056978172, -0.0066131437036356724, -0.006603227715641888, -0.006619809014489876, -0.006637559433675894, -0.006641227315996775, -0.006660618587849347, -0.00666995188974873, -0.006690555011193204, -0.0067030006510231934, -0.006703442904355629, -0.006719465886466936, -0.0067234507073410015, -0.006755913973065002, -0.0067754843008012286, -0.006777722624710781, -0.0067944643741339765, -0.006820241434285802, -0.0068157593342197675, -0.006838686939034971, -0.0068549042917204275, -0.006862586634799559, -0.006870751427594278, -0.006876373451233861, -0.006893173588203051, -0.006904185229225566, -0.006901171599177429, -0.006922926971321478, -0.006938050006805715, -0.006940696141516151, -0.006966623869397792, -0.006971895412029789, -0.006981021259016155, -0.007009362109027984, -0.007025897503720618, -0.007037267583709752, -0.007049290658795207, -0.007071266843540984, -0.00708712495272577, -0.007100888073132768, -0.007134093271505917, -0.007141149948828104, -0.007171452948710272, -0.007191172031964716, -0.007216233485587896]}, {[46.762, 47.022, 47.27, 47.517, 47.768, 48.03, 48.278, 48.522, 48.777, 49.026, 49.27, 49.522, 49.772, 50.025, 50.288, 50.534, 50.8, 51.05, 51.303, 51.563, 51.816, 52.08, 52.341, 52.605, 52.863, 53.113, 53.366, 53.624, 53.877, 54.135, 54.389, 54.652, 54.907, 55.16, 55.425, 55.68, 55.936, 56.19, 56.46, 56.719, 56.975, 57.228, 57.492, 57.746, 58.001, 58.265, 58.52, 58.774, 59.032, 59.296, 59.551, 59.801, 60.051, 60.311, 60.562, 60.813, 61.064, 61.32, 61.568, 61.816, 62.07, 62.319, 62.573, 62.819, 63.082, 63.334, 63.583, 63.836, 64.094, 64.347, 64.593, 64.857, 65.106, 65.358, 65.61, 65.87, 66.118, 66.367, 66.614, 66.87, 67.115, 67.36, 67.606, 67.859, 68.106, 68.352, 68.611, 68.86, 69.107, 69.355, 69.61, 69.857, 70.103, 70.35, 70.606, 70.853, 71.098, 71.348, 71.605, 71.853, 72.102, 72.356, 72.599, 72.844, 73.085, 73.338, 73.581, 73.825, 74.071, 74.329, 74.572, 74.815, 75.068, 75.315, 75.558, 75.803, 76.056, 76.3, 76.545, 76.787, 77.041, 77.284, 77.53, 77.779, 78.034, 78.279, 78.524, 78.778, 79.023, 79.265, 79.507, 79.759, 80.003, 80.245, 80.484, 80.741, 80.981, 81.226, 81.481, 81.722, 81.962, 82.202, 82.45, 82.69, 82.928, 83.167, 83.417, 83.662, 83.903, 84.147, 84.401, 84.644, 84.887, 85.141, 85.389, 85.635, 85.884, 86.14, 86.39], [0.002086772696673834, 0.0020895687873935197, 0.002074146352727511, 0.002064753043295853, 0.002053272792767245, 0.0020487518200479576, 0.002040094841932153, 0.0020369581512844313, 0.0020266241913334594, 0.0020174839473977506, 0.0020097555147348903, 0.0020057769200184554, 0.0019945100784537055, 0.001990526230713025, 0.0019827820308154307, 0.001979458045695198, 0.0019797255688577832, 0.001969401154420774, 0.001968273800180481, 0.0019567998381173615, 0.0019512917632464916, 0.0019479228081425214, 0.0019416327334357028, 0.001932175929685945, 0.0019331448859228756, 0.0019246564260766111, 0.0019191172155604706, 0.0018957350016240964, 0.0018985709931155798, 0.0018900891489435497, 0.0018701816054601784, 0.0018812704319993731, 0.001886520911460868, 0.0018391660814222664, 0.001856623350399602, 0.001847555991294646, 0.0018292168053281662, 0.0018450733984542833, 0.0018141657260208636, 0.0018058132968345104, 0.001795816361254391, 0.0017875992258848663, 0.00179191082819524, 0.0017811202920454037, 0.0017552279685040697, 0.001758648612648694, 0.0017240166134417523, 0.0017360682173226092, 0.0017285921409211367, 0.0017028007741323112, 0.0017019709665507554, 0.0016948875486640668, 0.0016747134137882482, 0.0016591658563382408, 0.0016421047721155737, 0.001631984656340071, 0.0016086992573891964, 0.0015995245512599196, 0.0016026983808973547, 0.0015967781374032137, 0.0015962693806482139, 0.001606045029976965, 0.001611396606119906, 0.0016086972370995259, 0.0015918792661511077, 0.0016109929594860294, 0.0015941249569382536, 0.0016018056234017558, 0.001593491686053143, 0.0016027887095701717, 0.001608373121547169, 0.0016101520104062827, 0.0016134974522765398, 0.0016151075161850842, 0.0016180001475377761, 0.0016192850841149978, 0.001620456202752229, 0.0015987051966247418, 0.0015985923370612208, 0.0016109115573409185, 0.0016115996711443432, 0.0016094368721478944, 0.0016007404945705928, 0.0016110405326884682, 0.0016119252520437936, 0.0016045959660831617, 0.0016109318031745704, 0.0015996470049593928, 0.0016043328825598934, 0.0016030896870392168, 0.0016126142065591804, 0.0016087125873794144, 0.0016061352576047863, 0.0016133276318860057, 0.001616779519748105, 0.0016270994739660042, 0.0016193394099180804, 0.0016232442798162507, 0.0016247910758278748, 0.0016231470755967035, 0.001626217080138835, 0.001626587929634265, 0.0016266385710323348, 0.0016306806116020583, 0.0016348140411213171, 0.0016363448554388487, 0.0016430697949435312, 0.0016480804346687584, 0.0016424508935514088, 0.0016457541569171927, 0.0016535975012183372, 0.0016540654197583651, 0.0016598418787008402, 0.0016688809186455914, 0.0016714202788960925, 0.001674011215317079, 0.0016803549984258672, 0.0016776731676202614, 0.0016810573981822807, 0.0016806256071464898, 0.0016849097329904225, 0.0016903222178388975, 0.0016909516502045911, 0.0016913173873336215, 0.0016975572791081506, 0.0016992916707921364, 0.001700350147736179, 0.0017027198554385268, 0.0017066723742497829, 0.0017069792769768468, 0.001714447393948102, 0.0017143392331105103, 0.001720950049921113, 0.0017243643671572748, 0.001723437726796853, 0.0017234769929865778, 0.001724743147334091, 0.001731494378238963, 0.001726768054316357, 0.0017318924316315945, 0.0017332650038122473, 0.0017286856973386198, 0.0017309308384353345, 0.0017390385254857366, 0.0017377630709113478, 0.0017409959943330852, 0.001744022398699889, 0.001746180512865643, 0.001747039801338161, 0.0017508941739130598, 0.0017578519004743736, 0.0017573213061995057, 0.0017624562960275821, 0.0017643207549933107, 0.0017646432721160107, 0.0017715099582221656, 0.0017692313591025982, 0.0017714767688185842, 0.0017784760587017446]}, {[46.762, 47.022, 47.27, 47.517, 47.768, 48.03, 48.278, 48.522, 48.777, 49.026, 49.27, 49.522, 49.772, 50.025, 50.288, 50.534, 50.8, 51.05, 51.303, 51.563, 51.816, 52.08, 52.341, 52.605, 52.863, 53.113, 53.366, 53.624, 53.877, 54.135, 54.389, 54.652, 54.907, 55.16, 55.425, 55.68, 55.936, 56.19, 56.46, 56.719, 56.975, 57.228, 57.492, 57.746, 58.001, 58.265, 58.52, 58.774, 59.032, 59.296, 59.551, 59.801, 60.051, 60.311, 60.562, 60.813, 61.064, 61.32, 61.568, 61.816, 62.07, 62.319, 62.573, 62.819, 63.082, 63.334, 63.583, 63.836, 64.094, 64.347, 64.593, 64.857, 65.106, 65.358, 65.61, 65.87, 66.118, 66.367, 66.614, 66.87, 67.115, 67.36, 67.606, 67.859, 68.106, 68.352, 68.611, 68.86, 69.107, 69.355, 69.61, 69.857, 70.103, 70.35, 70.606, 70.853, 71.098, 71.348, 71.605, 71.853, 72.102, 72.356, 72.599, 72.844, 73.085, 73.338, 73.581, 73.825, 74.071, 74.329, 74.572, 74.815, 75.068, 75.315, 75.558, 75.803, 76.056, 76.3, 76.545, 76.787, 77.041, 77.284, 77.53, 77.779, 78.034, 78.279, 78.524, 78.778, 79.023, 79.265, 79.507, 79.759, 80.003, 80.245, 80.484, 80.741, 80.981, 81.226, 81.481, 81.722, 81.962, 82.202, 82.45, 82.69, 82.928, 83.167, 83.417, 83.662, 83.903, 84.147, 84.401, 84.644, 84.887, 85.141, 85.389, 85.635, 85.884, 86.14, 86.39], [-0.002920105633059907, -0.002911042011710146, -0.0029067312952050983, -0.0028931818627671102, -0.002887028225511674, -0.002875850596681287, -0.002867127645044442, -0.002860596180655341, -0.0028532688911680794, -0.0028467048848256084, -0.0028356779770172947, -0.0028322589148603037, -0.002817847369034219, -0.002817554097238319, -0.002804144839777933, -0.002799384577849513, -0.002799169211173172, -0.002795769399417789, -0.002783978171847537, -0.0027739483333342, -0.002764788476245567, -0.002765949962456768, -0.002751693208201932, -0.002744579057626859, -0.002744721293363434, -0.002731345458488806, -0.0027270578907913723, -0.0027009941749409692, -0.00270384494611827, -0.0026916221945589656, -0.0026622851860537795, -0.0026814286412196247, -0.0026972389628016577, -0.0026458186577657935, -0.0026706578005200638, -0.002666136803189702, -0.0026400389342862355, -0.002680340997556137, -0.002651798601434968, -0.0026457781549903813, -0.0026446989218452707, -0.002640026334375809, -0.0026638603675147865, -0.002665451856561676, -0.002638907122103034, -0.002659690471530675, -0.002622929679255245, -0.00266795429340543, -0.0026684024466332884, -0.0026471224706954197, -0.0026681870637377406, -0.0026684774652430913, -0.0026683911349012226, -0.002667388466627868, -0.0026665490021019946, -0.002662945491287984, -0.0026571219589179296, -0.002653007332485728, -0.002648091384790765, -0.0026276803351357268, -0.0026235231766695843, -0.0026466802782904235, -0.0026437611596445113, -0.002646929128864437, -0.002615370393937268, -0.0026356299544573673, -0.0026173977280434355, -0.002634043665265642, -0.00261158000910025, -0.002631811161180919, -0.0026296103978386515, -0.002625976861680363, -0.002620287013979291, -0.002618466611762461, -0.0026183013936568814, -0.0026189433050958356, -0.0026228214156477367, -0.002600062815149793, -0.0025967224917708242, -0.002611390519069434, -0.0026124753069085745, -0.0026145985188550554, -0.002591233340690391, -0.002607907504566008, -0.0026032879582724654, -0.002607829700092668, -0.002608306794023655, -0.0025842605806546096, -0.002582898152640037, -0.0025837951833106894, -0.002587485440681786, -0.0025871161095297255, -0.002588987997303022, -0.0025854515193729894, -0.0025821672083031245, -0.0026147834920628487, -0.00259810368699632, -0.0026052284172718935, -0.0026116358514881744, -0.002614726483581838, -0.002618117508713452, -0.002624082476028249, -0.002632033527787018, -0.0026275871897094107, -0.002631241795640718, -0.0026312669243803216, -0.002629580022330731, -0.0026284420647624883, -0.0026213314037369312, -0.002622789487386972, -0.002625142726573219, -0.0026244281822515726, -0.002628968524820286, -0.0026249276908756132, -0.002622955733710297, -0.0026293957276682265, -0.002625006710368315, -0.0026292564575205813, -0.00263581521364536, -0.002636438509440678, -0.002641087006460176, -0.002645450735265452, -0.0026526276836859415, -0.002656381371643735, -0.0026566344650649997, -0.002661974950367707, -0.002663786907661198, -0.0026763327887088482, -0.002685146488934563, -0.002686191303104254, -0.002692720659100996, -0.002701069624310053, -0.0026990188729523836, -0.002707158010857917, -0.002714632659746611, -0.002714288518365523, -0.00271722973355451, -0.0027193452156867716, -0.0027237217409716605, -0.0027278143535760906, -0.0027275595436955305, -0.0027358252180669446, -0.0027400982402858297, -0.002743602606876035, -0.0027520316792993276, -0.002754860066732596, -0.0027581313859205868, -0.0027694734961789514, -0.002775844042533339, -0.002779809539337558, -0.0027856681364638505, -0.002795239009487128, -0.0028033911791087458, -0.0028106368885801323, -0.002823685546987438, -0.0028280509128323166, -0.0028399792516265224, -0.00284869435352031, -0.002859825099398711]}, {[46.762, 47.022, 47.27, 47.517, 47.768, 48.03, 48.278, 48.522, 48.777, 49.026, 49.27, 49.522, 49.772, 50.025, 50.288, 50.534, 50.8, 51.05, 51.303, 51.563, 51.816, 52.08, 52.341, 52.605, 52.863, 53.113, 53.366, 53.624, 53.877, 54.135, 54.389, 54.652, 54.907, 55.16, 55.425, 55.68, 55.936, 56.19, 56.46, 56.719, 56.975, 57.228, 57.492, 57.746, 58.001, 58.265, 58.52, 58.774, 59.032, 59.296, 59.551, 59.801, 60.051, 60.311, 60.562, 60.813, 61.064, 61.32, 61.568, 61.816, 62.07, 62.319, 62.573, 62.819, 63.082, 63.334, 63.583, 63.836, 64.094, 64.347, 64.593, 64.857, 65.106, 65.358, 65.61, 65.87, 66.118, 66.367, 66.614, 66.87, 67.115, 67.36, 67.606, 67.859, 68.106, 68.352, 68.611, 68.86, 69.107, 69.355, 69.61, 69.857, 70.103, 70.35, 70.606, 70.853, 71.098, 71.348, 71.605, 71.853, 72.102, 72.356, 72.599, 72.844, 73.085, 73.338, 73.581, 73.825, 74.071, 74.329, 74.572, 74.815, 75.068, 75.315, 75.558, 75.803, 76.056, 76.3, 76.545, 76.787, 77.041, 77.284, 77.53, 77.779, 78.034, 78.279, 78.524, 78.778, 79.023, 79.265, 79.507, 79.759, 80.003, 80.245, 80.484, 80.741, 80.981, 81.226, 81.481, 81.722, 81.962, 82.202, 82.45, 82.69, 82.928, 83.167, 83.417, 83.662, 83.903, 84.147, 84.401, 84.644, 84.887, 85.141, 85.389, 85.635, 85.884, 86.14, 86.39], [-0.0029942919853128934, -0.002981232675787013, -0.002981605522587964, -0.0029720974695458904, -0.002968111538032384, -0.002957229069180692, -0.0029519873097402717, -0.0029432644292471354, -0.0029354101234494185, -0.0029323538956400135, -0.0029223854192257696, -0.002921156247958574, -0.0029081432484259124, -0.002907888948838728, -0.0028982746418024456, -0.00289433166273525, -0.0028954687088156798, -0.0028951781024710707, -0.002880459745563115, -0.0028741353494116965, -0.002866384727359443, -0.0028712113787737904, -0.002854736345435376, -0.00285237699387285, -0.0028537044442461827, -0.002842172600940781, -0.0028424546043804367, -0.00281518168749209, -0.0028178377315482652, -0.0028066637063588694, -0.0027748684070497253, -0.0027982293458960273, -0.0028213394729748706, -0.0027707848304051722, -0.002796813060678673, -0.0027979166480531534, -0.002775475176605448, -0.0028239654719128117, -0.002800269194112849, -0.0027988611041543108, -0.0028060521461332304, -0.0028079761257325613, -0.002842125642980982, -0.0028553604063332547, -0.0028358136112332853, -0.002867753024683733, -0.0028409843692267156, -0.002902234210220969, -0.002915599693240355, -0.002903731914194381, -0.0029397008907958984, -0.0029515439431981746, -0.002967165422917084, -0.002978569566597687, -0.0029897314368889467, -0.0029987549345562563, -0.0030071013001323286, -0.0030120666834490663, -0.0029966578775210357, -0.002962740122176991, -0.002950921883849161, -0.0029715265194784034, -0.002963100833106865, -0.0029662424471492694, -0.0029265370860368668, -0.002945960659451683, -0.002924348157761158, -0.002941041684131702, -0.0029106941846051915, -0.0029306295175145786, -0.002924795083939522, -0.0029165840743613117, -0.0029053410420472924, -0.002902355554655587, -0.002896745671189564, -0.0028918537633711517, -0.0028936939809043253, -0.0028674490197746058, -0.002861283769695954, -0.0028718802448856797, -0.002868489306398771, -0.0028678553138846647, -0.002838576898339344, -0.002852103087663805, -0.0028441003894435616, -0.002847253918290718, -0.00284295424625466, -0.0028110129649790597, -0.002805788907181798, -0.0028043349316880495, -0.0028054153090983965, -0.002803932872982209, -0.002805910343268356, -0.002798066441978025, -0.002792893333732718, -0.002828252302803895, -0.002809184909778639, -0.0028150390003046457, -0.002821483260438551, -0.002824825067715257, -0.0028291697443978323, -0.0028328997080085375, -0.0028415687993638855, -0.002834375727720802, -0.0028382039175843267, -0.0028314723762046952, -0.00282900861967338, -0.0028216733049318656, -0.002811901818184866, -0.0028112105533878813, -0.0028096264904133683, -0.0027994731245004536, -0.002802251660182127, -0.0027958750159070276, -0.0027907032434500356, -0.002792456925628432, -0.0027844780191294155, -0.002786819300324688, -0.0027932271391257874, -0.0027929080712978302, -0.00279292363377571, -0.002797620687557768, -0.0028047747177899424, -0.0028074647144746916, -0.002805960011438999, -0.0028104379107938325, -0.0028125637476831885, -0.002826845149032929, -0.0028378351920827155, -0.0028389874805839696, -0.002844822193146778, -0.0028524588561001083, -0.0028475559020575297, -0.0028550064637021, -0.002865717532207256, -0.0028603680274402006, -0.0028632467898694423, -0.0028636763511668034, -0.002866762224035284, -0.002870163155142264, -0.002870455796364166, -0.0028811686680646907, -0.002883273643173954, -0.002889059474542748, -0.0028968445033299506, -0.0029003084709092056, -0.00290290560034323, -0.0029163196064853213, -0.002923392603090001, -0.0029263999886074703, -0.0029331641316016977, -0.0029459898565634287, -0.00295713815561183, -0.0029678403129062467, -0.002983545887626406, -0.0029889815657189196, -0.0030040972523025186, -0.0030153071374456712, -0.0030287682559420794]}, {[46.762, 47.022, 47.27, 47.517, 47.768, 48.03, 48.278, 48.522, 48.777, 49.026, 49.27, 49.522, 49.772, 50.025, 50.288, 50.534, 50.8, 51.05, 51.303, 51.563, 51.816, 52.08, 52.341, 52.605, 52.863, 53.113, 53.366, 53.624, 53.877, 54.135, 54.389, 54.652, 54.907, 55.16, 55.425, 55.68, 55.936, 56.19, 56.46, 56.719, 56.975, 57.228, 57.492, 57.746, 58.001, 58.265, 58.52, 58.774, 59.032, 59.296, 59.551, 59.801, 60.051, 60.311, 60.562, 60.813, 61.064, 61.32, 61.568, 61.816, 62.07, 62.319, 62.573, 62.819, 63.082, 63.334, 63.583, 63.836, 64.094, 64.347, 64.593, 64.857, 65.106, 65.358, 65.61, 65.87, 66.118, 66.367, 66.614, 66.87, 67.115, 67.36, 67.606, 67.859, 68.106, 68.352, 68.611, 68.86, 69.107, 69.355, 69.61, 69.857, 70.103, 70.35, 70.606, 70.853, 71.098, 71.348, 71.605, 71.853, 72.102, 72.356, 72.599, 72.844, 73.085, 73.338, 73.581, 73.825, 74.071, 74.329, 74.572, 74.815, 75.068, 75.315, 75.558, 75.803, 76.056, 76.3, 76.545, 76.787, 77.041, 77.284, 77.53, 77.779, 78.034, 78.279, 78.524, 78.778, 79.023, 79.265, 79.507, 79.759, 80.003, 80.245, 80.484, 80.741, 80.981, 81.226, 81.481, 81.722, 81.962, 82.202, 82.45, 82.69, 82.928, 83.167, 83.417, 83.662, 83.903, 84.147, 84.401, 84.644, 84.887, 85.141, 85.389, 85.635, 85.884, 86.14, 86.39], [-0.0019226244373978954, -0.0019212488086039498, -0.0019153313525979568, -0.0019138642557726413, -0.0019085988040364065, -0.0019039617797162183, -0.0019035070604725606, -0.001900688750941829, -0.0018885111266778458, -0.0018842512480821592, -0.0018828330679168126, -0.001880246705922257, -0.0018740240860696472, -0.001870343767072435, -0.0018692010728406136, -0.001867437237591872, -0.0018687147585050826, -0.0018631209274937663, -0.0018567315865805512, -0.0018508428928338536, -0.0018499501911031207, -0.001848617209868317, -0.001843079706895622, -0.0018442717738304663, -0.001844495448558146, -0.00184256253378063, -0.0018402633391694117, -0.0018153088692980065, -0.0018200750772611905, -0.0018134177464901458, -0.001794278757683699, -0.0018087660523015095, -0.001821831259349332, -0.001776968124000837, -0.0017932719596787364, -0.0017932831574255254, -0.0017811453540617314, -0.0018069893886549638, -0.0017815295119909412, -0.0017804503678592234, -0.0017789038607723272, -0.0017809292562655013, -0.0017975796825003157, -0.0018017152617011277, -0.0017837642058920005, -0.0017999640848161513, -0.0017772498825691639, -0.0018058760574106156, -0.0018135936879222654, -0.001798452991561441, -0.0018113915264740522, -0.0018189859380058704, -0.0018123555642463028, -0.0018090051063063292, -0.0018058478464062645, -0.0018118717692831062, -0.0018060113003346215, -0.0018116340662311203, -0.0018060547801411373, -0.0017894418161260573, -0.0017821851356272782, -0.0017864138590434455, -0.001791214976629817, -0.0017883271002048606, -0.0017621337418264524, -0.0017842985008644874, -0.001763443444937926, -0.0017751486151926974, -0.0017620186081212343, -0.0017702289646113285, -0.0017764346866753265, -0.0017741690032581944, -0.0017770874752413323, -0.0017802891817591863, -0.001778224725189678, -0.0017759598457293274, -0.0017763999783206015, -0.0017512067317826622, -0.0017525335950286617, -0.0017609211027336958, -0.0017576778354439124, -0.0017524207271604883, -0.0017420363742623591, -0.0017491822012112176, -0.0017480011719624119, -0.0017381614761900288, -0.0017411250676089899, -0.001728507988856727, -0.001732156306654929, -0.0017290108332126742, -0.0017383891982339138, -0.0017342722445094344, -0.0017316136153277114, -0.0017394358189098754, -0.0017441000729392197, -0.0017549307474527716, -0.0017470277320761017, -0.0017512163896778023, -0.0017526387177197744, -0.0017515082445692467, -0.0017580329705569721, -0.001756665085264172, -0.0017565766061356852, -0.0017620228084034852, -0.0017681572925431566, -0.0017630043888548776, -0.0017726191670218306, -0.001771512438981266, -0.001764273288361736, -0.0017655639964531066, -0.0017724738646714366, -0.0017675627904639166, -0.0017725983139348501, -0.0017844397869895164, -0.001786903584969244, -0.0017858736146308435, -0.0017931123927769602, -0.001789052105129971, -0.0017923843716966023, -0.0017907924124746387, -0.0017920965976447904, -0.0017999063938516145, -0.00179984427721216, -0.001799541908515084, -0.0018078265894014725, -0.001809478193303419, -0.0018120632652024187, -0.0018146315683952156, -0.0018226592855806868, -0.0018252808085356972, -0.0018330755464399753, -0.0018302074503218672, -0.0018379909404393122, -0.0018422867703653551, -0.0018448144452243576, -0.0018401607554953488, -0.0018408778498601366, -0.001849028367988376, -0.001843101573025602, -0.001846958952606333, -0.001852519389884004, -0.0018488131039057414, -0.0018491714323448916, -0.0018601405434676896, -0.0018583021168365342, -0.0018642671394345659, -0.0018677446634936337, -0.0018711700235951563, -0.0018738940621950589, -0.0018774902272286425, -0.0018873234444391578, -0.001890684104904851, -0.001900156968597599, -0.0019069431360274885, -0.0019080932698261948, -0.0019199858613651805, -0.0019181884393049333, -0.001923449140878496, -0.0019330455322994842]}]
  out "Plot:   optimal subspace":cluster{dbl[], dbl[]}[](graph)=[{[55.393, 55.473, 55.549, 55.623, 55.697, 55.77, 55.847, 55.926, 56.007, 56.087, 56.169, 56.251, 56.332, 56.409, 56.489, 56.565, 56.645, 56.724, 56.8, 56.877, 56.955, 57.034, 57.114, 57.191, 57.269, 57.348, 57.425, 57.505, 57.583, 57.656, 57.736, 57.815, 57.896, 57.974, 58.055, 58.137, 58.217, 58.295, 58.373, 58.45, 58.526, 58.605, 58.679, 58.759, 58.836, 58.913, 58.989, 59.071, 59.148, 59.226, 59.302, 59.381, 59.459, 59.539, 59.616, 59.694, 59.77, 59.846, 59.925, 59.998, 60.076, 60.154, 60.23, 60.308, 60.384, 60.462, 60.54, 60.618, 60.693, 60.77, 60.849, 60.928, 61.004, 61.082, 61.16, 61.239, 61.315, 61.391, 61.468, 61.544, 61.626, 61.703, 61.781, 61.86, 61.93, 62.009, 62.083, 62.162, 62.238, 62.312, 62.389, 62.466, 62.541, 62.618, 62.697, 62.774, 62.854, 63.013, 63.088, 63.165, 63.241, 63.317, 63.394, 63.472, 63.549, 63.628, 63.705, 63.782, 63.861, 63.937, 64.014, 64.089, 64.162, 64.239, 64.316, 64.393, 64.47, 64.547, 64.62, 64.696, 64.817, 64.892, 64.971, 65.046, 65.123, 65.2, 65.275, 65.35, 65.429, 65.507, 65.582, 65.655, 65.733, 65.81, 65.887, 65.965, 66.042, 66.193, 66.27, 66.345, 66.423, 66.5, 66.574, 66.651, 66.728, 66.802, 66.881, 66.956, 67.032, 67.108, 67.187, 67.258, 67.335, 67.411, 67.487, 67.563, 67.639, 67.717, 67.792, 67.869, 67.941, 68.018, 68.097, 68.174, 68.251, 68.349, 68.484, 68.558, 68.632, 68.708, 68.787, 68.864, 69.014, 69.092, 69.169, 69.246, 69.323, 69.397, 69.472, 69.546, 69.621, 69.696, 69.771, 69.845, 69.924, 69.997, 70.071, 70.149, 70.225, 70.301, 70.381, 70.457, 70.533, 70.609, 70.682, 70.76, 70.84, 70.915, 70.993, 71.145, 71.222, 71.3, 71.374, 71.452], [-0.6539993268930167, 0.3391236144564683, -0.09456432043806404, 0.0051367164973633896, 0.0020044244170662685, 0.011874272381953276, 0.06955451759566218, 0.007725271948397916, -0.004046329903722955, 0.012996231366623931, 0.02336389200775809, 0.024693616597254348, -0.043124477823421006, -0.017775933941850515, 0.04206965874272625, -0.11798708971321988, -0.08203489517148861, 0.015852951226723568, -0.06159173734444465, -0.0906144627663518, -0.048921335123773224, -0.025097551631409025, 0.03747376904568885, 0.026314885922756725, -0.08142107802798851, -0.04367395508948556, 0.025063497548666342, 0.037473769045688714, -0.09061446276635161, 0.07028982367908473, -0.037287084745676984, -0.03331452126771534, -0.0014293476377641413, -0.0291901136218296, 0.0446928180029198, 0.00290562753315699, 0.012066348733460198, 0.012562461680758148, -0.018476184956469036, 0.024652499530850507, -0.00011169769376606508, -0.043673955089485336, -0.034237925342999874, -0.041796842880443226, 0.03260096402459978, 0.013337833923163239, 0.028074032981141733, 0.02479303749859956, 0.04773146565334352, -0.0917979629943126, -0.08210132900667996, 0.07469329051450514, 0.04284862090477776, -0.048649980732486074, 0.05107537884702248, -0.045809372663442795, 0.12325677070152805, 0.05609768493174689, -0.002976243880241466, 0.055086131759920394, -0.010877679296898951, -0.029218379981849323, -0.010877679296900285, -0.048682509171851414, -0.08284375332862261, 0.11159983091108487, -0.02061373332521245, 0.07830420438142319, -0.05749858935992324, 0.030209847921128213, 0.033187881765827563, 0.0632454769770712, 0.011685909194376521, 0.014141087261257316, 0.09595339373441054, 0.034766252436734583, -0.06982174337419339, -0.0082770012246038, -0.02630887225081902, -0.09198148956369846, 0.011620057966691983, 0.012656148379396237, 0.02704444806042294, -0.055089665311336876, -0.010877679296900226, 0.11265218201672413, -0.027770881489970173, 0.014843280637345453, -0.023190740122303075, 0.057998283736627604, 0.025404299712243082, 0.05096886575937984, -0.011041283301146457, -0.0785294557445813, -0.1179870897132201, 0.01825031298729252, 0.004059220722186789, 0.009722439156744988, 0.06360381321170706, -0.03557589423855971, -0.03658151530191978, -0.059497458408195626, -0.019694269436186972, 0.07525056135337402, -0.04945967745638282, 0.02704444806042326, -0.023748803061154487, 0.054380122215328834, -0.07703437213244521, 0.08566875796505154, -0.020251331993503582, -0.023952284418691773, -0.02952998594490326, 0.04206965874272611, 0.015136067978359483, -0.07102312521130782, 0.04110574188038118, -0.047734799331777364, -0.009159302165546394, 0.05123083050100717, 0.16247491505060013, -0.03658151530191925, -0.04055517231337933, -0.06397759432387508, 0.05000696501163893, -0.02274052786555141, -0.036117801828781416, 0.06438911827431076, -0.06397759432387551, 0.07902148482902957, 0.07091125409732564, 0.05660232490132762, 0.003488096034465255, 0.06098287440769287, -0.07312812028096935, -0.03997679857564285, 0.06966129911814035, -0.01200735338094387, 0.0011683041305290498, -0.026973944618607863, 0.014809638246185298, 0.05660232490132767, -0.042969630453861575, -0.0008353715209700875, -0.009143131205386776, 0.04385368363874332, 0.03122354997581172, 0.023208866857712538, -0.011927566069049402, 0.011685909194375446, 0.01752271351681508, -0.016581982918802186, 0.014945230605948495, 0.00875427084575472, 0.03168710415197408, -0.01658087713761681, -0.006730271771716752, -0.006780822682695883, -0.04222734411828173, 0.0011683041305291441, 0.04477780338783405, 0.016848841839736322, 0.024236387665468876, 0.011563814441528143, 0.08814160730020291, 0.023632730480340702, -0.019314907742346392, 0.023208866857712732, 0.01770600216283244, 0.0034828877704507445, -0.030412875700733543, 0.02234017525324682, -0.04617557628949561, -0.06294948272567681, -0.009373798802334287, 0.026878262977207832, -0.052669278619909915, -0.0038344873940750553, 0.02897704740047952, 0.0040978082744671795, 0.04452617477957913, -0.11255781245377125, 0.04010898135209824, 0.0610473165358694, 0.02223933544743438, 0.02241750520192594, -0.007179708450721197, 0.0014508139903299858, 0.02491818912257842, -0.013717635945350942, 0.02357438582599947, 0.028669025739076148, 0.0536097823579598, -0.001068008136356144, 0.038631164135670075, -0.012463770264631075, 0.01336088595160985, 0.012451807078451239, -0.03804059074580767, 0.010373724593344768, 0.025629310861148537, -0.0053638644795241846, -0.012735855163042972, -0.05318586105391781]}, ...(2 in all)]
  out "element":i32=1904
  out "min T":dbl=55.39488157894737
  out "max T":dbl=71.55988157894737
  out "Array of dL":dbl[][](array[numeric])=[[0.02755377978914764, -0.05, 0.08, 0.34, 0.03244622021085236, 0.25], [-0.14203417026277648, -0.06, 0.11, 0.16, 0.15203417026277652, 0.29], [-0.19497344643867404, -0.15, 0.1, 0.58, 0.2549734464386741, 0.0], [0.2303603238799098, -0.21, 0.19, 0.17, 0.0496396761200902, 0.29]]
  out "peaks -- used":i32[](array[numeric])=[1904]
  out "Array of eigenvalues":dbl[](array[numeric])=[3.904083486932411e-15, 405.5406354503157]
  in  "dimension":i32=2
  in  "gauge: offset":dbl(slide)=1e-09 min=1e-09 max=10.0 step=1e-08 scale=1e-09..10.0 scale format="%#_2g"
  in  "averaging window":i32(slide) min=0 max=50 step=1 scale=0.01..50.0
  out "subarray":dbl[](array[numeric])=[0.02755377978914764, -0.05, 0.08, 0.34, 0.03244622021085236, 0.25]
  out "String":string=" 1904, "
  in  "read/write buttons":T2[](array[typedef])=[{"Boolean"=FALSE, "String"="read buttons"}, {"Boolean"=FALSE, "String"="write buttons"}]
  in  "what query":T2[](array[typedef])=[{"Boolean"=FALSE, "String"="frequency"}, {"Boolean"=FALSE, "String"="attenuation"}, {"Boolean"=FALSE, "String"="deltafreq"}, {"Boolean"=FALSE, "String"="Vardeltafreq"}, {"Boolean"=FALSE, "String"="log 1/Q"}, {"Boolean"=FALSE, "String"="1/Q"}, {"Boolean"=FALSE, "String"="norm. attenuation"}, {"Boolean"=TRUE, "String"="log gamma"}, {"Boolean"=FALSE, "String"="VarDeltaFreq div f"}]
  in  "sweep folder path":path=path "E:/data/Ultrasound/Experiment/ProbeTest/Probe10/YBCO_5/sweep5"
  in  "temperature mapping":T2[](array[typedef])=[{"Boolean"=FALSE, "String"="read buttons"}, {"Boolean"=FALSE, "String"="write buttons"}]
  in  "what 2":T3(ring)=enum."log gamma"
  in  "linear residue?":enum16{"linear", "quadratic", "nothing"}(ring)=enum."nothing"
  in  "residue?":bool
  out "K per min":dbl
  out "# of peaks":i32=1
  out "# of temperatures":i32=204
  out "number of rows":i32=4
  out "number of columns":i32=159
  out "number of rows 2":i32=6
  out "number of columns 2":i32=4
  out "number of rows 3":i32=6
  out "number of columns 3":i32=159
  in  "array of coefficients":dbl[][](array[numeric])=[[5.0, 7.0, -1.75, 2.796875, 3.0, 1.875], [-5.5, -5.5, -2.0, -1.71875, -2.0, 2.75], [1.0, -0.5, 2.0, 0.78125, 3.0, -1.25], [1.5, -3.0, 3.25, -0.671875, 0.5, -0.375]]
  out "size(s)":i32[](array[numeric])=[4, 6]
  in  "cursor bracket: All, data window":T4={"left"=55.39488157894737, "right "=71.55988157894737, "center"=61.05263157894737, "window"=16.165, "cursors"=[0, 1, 2], "relative"=1, "absolute"=1, "fixed vertical offset"=0.0, "vertical offset"=0.0, "skew"=0.0, "default window frac"=0.3, "kind"=enum."symmetric", "skew.left"=0.5, "skew.right"=0.0, "Plot ref"=refnum, "wing order"=enum."back"}
  out "common temperature points":dbl[](array[numeric])=[55.393, 55.473, 55.549, 55.623, 55.697, 55.77, 55.847, 55.926, 56.007, 56.087, 56.169, 56.251, 56.332, 56.409, 56.489, 56.565, 56.645, 56.724, 56.8, 56.877, 56.955, 57.034, 57.114, 57.191, 57.269, 57.348, 57.425, 57.505, 57.583, 57.656, 57.736, 57.815, 57.896, 57.974, 58.055, 58.137, 58.217, 58.295, 58.373, 58.45, 58.526, 58.605, 58.679, 58.759, 58.836, 58.913, 58.989, 59.071, 59.148, 59.226, 59.302, 59.381, 59.459, 59.539, 59.616, 59.694, 59.77, 59.846, 59.925, 59.998, 60.076, 60.154, 60.23, 60.308, 60.384, 60.462, 60.54, 60.618, 60.693, 60.77, 60.849, 60.928, 61.004, 61.082, 61.16, 61.239, 61.315, 61.391, 61.468, 61.544, 61.626, 61.703, 61.781, 61.86, 61.93, 62.009, 62.083, 62.162, 62.238, 62.312, 62.389, 62.466, 62.541, 62.618, 62.697, 62.774, 62.854, 63.013, 63.088, 63.165, 63.241, 63.317, 63.394, 63.472, 63.549, 63.628, 63.705, 63.782, 63.861, 63.937, 64.014, 64.089, 64.162, 64.239, 64.316, 64.393, 64.47, 64.547, 64.62, 64.696, 64.817, 64.892, 64.971, 65.046, 65.123, 65.2, 65.275, 65.35, 65.429, 65.507, 65.582, 65.655, 65.733, 65.81, 65.887, 65.965, 66.042, 66.193, 66.27, 66.345, 66.423, 66.5, 66.574, 66.651, 66.728, 66.802, 66.881, 66.956, 67.032, 67.108, 67.187, 67.258, 67.335, 67.411, 67.487, 67.563, 67.639, 67.717, 67.792, 67.869, 67.941, 68.018, 68.097, 68.174, 68.251, 68.349, 68.484, 68.558, 68.632, 68.708, 68.787, 68.864, 69.014, 69.092, 69.169, 69.246, 69.323, 69.397, 69.472, 69.546, 69.621, 69.696, 69.771, 69.845, 69.924, 69.997, 70.071, 70.149, 70.225, 70.301, 70.381, 70.457, 70.533, 70.609, 70.682, 70.76, 70.84, 70.915, 70.993, 71.145, 71.222, 71.3, 71.374, 71.452]
  in  "cursor bracket: Plot:   what vs temp":T4={"left"=125.5, "right "=130.5, "center"=128.0, "window"=5.0, "cursors"=[0, 1, 2], "relative"=1, "absolute"=1, "fixed vertical offset"=0.0, "vertical offset"=0.0, "skew"=0.0, "default window frac"=0.3, "kind"=enum."skewed", "skew.left"=0.5, "skew.right"=1.0, "Plot ref"=refnum, "wing order"=enum."back"}
  out "temperature points OUT":dbl[](array[numeric])=[55.393, 55.473, 55.549, 55.623, 55.697, 55.77, 55.847, 55.926, 56.007, 56.087, 56.169, 56.251, 56.332, 56.409, 56.489, 56.565, 56.645, 56.724, 56.8, 56.877, 56.955, 57.034, 57.114, 57.191, 57.269, 57.348, 57.425, 57.505, 57.583, 57.656, 57.736, 57.815, 57.896, 57.974, 58.055, 58.137, 58.217, 58.295, 58.373, 58.45, 58.526, 58.605, 58.679, 58.759, 58.836, 58.913, 58.989, 59.071, 59.148, 59.226, 59.302, 59.381, 59.459, 59.539, 59.616, 59.694, 59.77, 59.846, 59.925, 59.998, 60.076, 60.154, 60.23, 60.308, 60.384, 60.462, 60.54, 60.618, 60.693, 60.77, 60.849, 60.928, 61.004, 61.082, 61.16, 61.239, 61.315, 61.391, 61.468, 61.544, 61.626, 61.703, 61.781, 61.86, 61.93, 62.009, 62.083, 62.162, 62.238, 62.312, 62.389, 62.466, 62.541, 62.618, 62.697, 62.774, 62.854, 63.013, 63.088, 63.165, 63.241, 63.317, 63.394, 63.472, 63.549, 63.628, 63.705, 63.782, 63.861, 63.937, 64.014, 64.089, 64.162, 64.239, 64.316, 64.393, 64.47, 64.547, 64.62, 64.696, 64.817, 64.892, 64.971, 65.046, 65.123, 65.2, 65.275, 65.35, 65.429, 65.507, 65.582, 65.655, 65.733, 65.81, 65.887, 65.965, 66.042, 66.193, 66.27, 66.345, 66.423, 66.5, 66.574, 66.651, 66.728, 66.802, 66.881, 66.956, 67.032, 67.108, 67.187, 67.258, 67.335, 67.411, 67.487, 67.563, 67.639, 67.717, 67.792, 67.869, 67.941, 68.018, 68.097, 68.174, 68.251, 68.349, 68.484, 68.558, 68.632, 68.708, 68.787, 68.864, 69.014, 69.092, 69.169, 69.246, 69.323, 69.397, 69.472, 69.546, 69.621, 69.696, 69.771, 69.845, 69.924, 69.997, 70.071, 70.149, 70.225, 70.301, 70.381, 70.457, 70.533, 70.609, 70.682, 70.76, 70.84, 70.915, 70.993, 71.145, 71.222, 71.3, 71.374, 71.452]
  out "what points out":dbl[](array[numeric])=[-1.4233131928950045, -1.44696698189356, -1.4387793191620561, -1.4336803765711887, -1.4766437914412072, -1.4238891039751602, -1.4266641580299324, -1.4249276723821875, -1.4343882731939412, -1.4156687737284692, -1.4512421695222957, -1.429807437000274, -1.4155556909308238, -1.4387793191620561, -1.4256214336829176, -1.4378261347313517, -1.472241245575028, -1.476513665752772, -1.4669909756005146, -1.430275048869841, -1.4314462860465573, -1.4375881651462725, -1.4885177094699984, -1.3721223035160284, -1.4390179425097644, -1.430626088480954, -1.4084901891013457, -1.4885177094699984, -1.430275048869841, -1.4816176825506562, -1.4117282912536708, -1.420102128492896, -1.414200989082999, -1.4412914275628341, -1.4275931305379441, -1.4362816581303222, -1.4294570582141024, -1.449038245797824, -1.4286406053421603, -1.431211785780653, -1.4307431647673898, -1.430626088480954, -1.4310945831131212, -1.4301580986922384, -1.4330913428691965, -1.5284149439108103, -1.450996736070212, -1.449404790606672, -1.4596705233051261, -1.4422522564545317, -1.4500163869363112, -1.4513649382812484, -1.4485500001231248, -1.4439388390864674, -1.4579218517603743, -1.4631891321044586, -1.465593098958123, -1.4559319537457243, -1.4673729968671088, -1.447210147903218, -1.447696888757646, -1.4348608461262105, -1.447696888757646, -1.4373503258840832, -1.438898614446944, -1.4737899942543355, -1.4484280244217462, -1.4242350175592806, -1.4386600566370986, -1.5039010059634286, -1.4487940543480937, -1.4347426546757862, -1.4293403280744659, -1.4346244953819263, -1.4560560556130935, -1.486382924308125, -1.4525945384285102, -1.5065419471008115, -1.4360445331001872, -1.4326206904450212, -1.4059390968255816, -1.4248121531683389, -1.4270122898977948, -1.4435768767247146, -1.447696888757646, -1.4271283958955197, -1.4268962149320088, -1.4462382997059955, -1.4219341142599085, -1.425968730368281, -1.438540826854084, -1.423773860646395, -1.4007721353222036, -1.4364002692144688, -1.4378261347313517, -1.4333268604898834, -1.4255057298106724, -1.4776862029393325, -1.4273607010531868, -1.4207882178645008, -1.4189610493238327, -1.42969061266012, -1.4112802184959434, -1.4282911662873123, -1.4605475065465392, -1.4270122898977948, -1.394479474658531, -1.4281747490551708, -1.4212462136695654, -1.4236586478902071, -1.407823240700133, -1.4039529905505608, -1.4082677591441644, -1.4256214336829176, -1.41016205494854, -1.4115041970887898, -1.413187728652624, -1.411840381712908, -1.404944908336696, -1.4094925360874166, -1.4263163050022019, -1.4189610493238327, -1.4191890254350537, -1.4124012683747549, -1.4031830621804093, -1.4027437151708582, -1.399462703731531, -1.4038429171798275, -1.4124012683747549, -1.4015377976218495, -1.3966390737476193, -1.4086014468147512, -1.3976144079908948, -1.398265849835895, -1.4081565868712154, -1.3873220797794983, -1.396206293959037, -1.4042833781525756, -1.3759242669503173, -1.3791355228308788, -1.384365529218584, -1.4086014468147512, -1.3885953603844066, -1.402633947829972, -1.3902988957166005, -1.3972890531384425, -1.400007820511902, -1.3731465834292742, -1.376440608090563, -1.4293403280744659, -1.3726341415032672, -1.3798639431222424, -1.3880643730558775, -1.3630108962837708, -1.3713046153819766, -1.392009139548825, -1.3360165434877334, -1.3750993958915096, -1.3514448424333292, -1.3759242669503173, -1.372224622866697, -1.3371477648312038, -1.3381873125587387, -1.3768541234580602, -1.3643152355487773, -1.3590219407376678, -1.3521282327897675, -1.3731465834292742, -1.3689623015592596, -1.3502758121664775, -1.3365817858433202, -1.3120253780614444, -1.3605135088274138, -1.3602147851091797, -1.3516399871150684, -1.3737623129490995, -1.35261702798138, -1.3653212459173176, -1.351835219521999, -1.3320803127786385, -1.372736581527779, -1.410608974959067, -1.3461124400250224, -1.4067139310755428, -1.308830063964396, -1.3486250541829568, -1.3950183684885684, -1.349304018335389, -1.3283644014938703, -1.3056580877318187, -1.3363932899714797, -1.3342314473766201, -1.3269790909671038, -1.3485281458969576, -1.3613111114058765, -1.3408447171553701, -1.330962197210844, -1.324863493628006, -1.3103360330802296, -1.3067128410903444, -1.3183969993651314, -1.3216637513638199, -1.32947584031392, -1.3245883043811366]
  in  "active buttons ref":refnum<vi>
  out "button list array":refnum<vi>[](array[refnum])
  out "rusout file":T5={"freqs Exp"=[0.56399, 0.64865, 0.98705, 1.13311, 1.21355, 1.58494, 1.7634, 1.82275, 1.88042, 1.89886, 2.03162, 2.13781, 2.22097, 2.27018, 2.34957, 2.45631, 2.58035, 2.63386, 2.83114, 2.9599, 2.96507, 3.13063, 3.32755, 3.46889, 3.55331, 0.0, 3.61506, 3.73397, 0.0, 0.0, 0.0, 4.23646, 4.3003, 4.33064], "symmetry"=[4, 6, 6, 2, 8, 1, 8, 5, 4, 3, 6, 7, 5, 2, 4, 5, 6, 7, 8, 2, 1, 2, 3, 6, 8, 6, 3, 4, 5, 1, 8, 7, 7, 4], "dc11"=[0.01, 0.41, 1.32, 0.07, 0.77, 0.2, 0.08, 0.94, 0.2, 0.03, 0.23, 1.68, 1.24, 1.15, 0.81, 1.17, 0.07, 0.79, 0.1, 0.3, 0.53, 0.27, 0.44, 0.71, 0.7, 0.24, 1.1, 0.23, 0.48, 0.7, 0.15, 0.3, 0.16, 0.09], "freqs Fit"=[0.550578, 0.652035, 0.99108, 1.161515, 1.272787, 1.59078, 1.643052, 1.818228, 1.931688, 1.95078, 2.000057, 2.071117, 2.16399, 2.176296, 2.418359, 2.556268, 2.69381, 2.74406, 2.786674, 2.851041, 2.888839, 3.072063, 3.182576, 3.500314, 3.595723, 3.658982, 3.675366, 3.705338, 3.761767, 3.812625, 3.852628, 3.891519, 3.946262, 3.978336], "header"=" LANL RPRcode Ver. 6.1\r ;YBCO_5    310K                         \r", "bulk modulus"=0.8473, "c11"=2.64179, "c22"=2.64775, "free moduli"=["c11", "c22", "c33", "c23", "c13", "c12", "c44", "c55", "c66"], "# of polynomials"=14, "mass, g"=0.0016, "density, g/cm3"=6.429, "dc22"=[0.02, 1.56, 0.1, 0.42, 0.24, 1.49, 1.04, 1.53, 0.72, 0.11, 0.1, 0.23, 0.85, 0.08, 0.08, 0.28, 0.92, 0.99, 0.23, 0.5, 0.44, 0.26, 0.72, 0.15, 0.26, 0.24, 1.29, 0.15, 0.76, 0.55, 0.53, 0.62, 1.12, 0.57], "dc33"=[0.01, 0.15, 0.56, 0.06, 0.1, 0.23, 0.34, 0.02, 0.07, 0.04, 0.09, 0.35, 0.36, 0.32, 0.26, 0.9, 0.2, 0.14, 0.08, 0.11, 0.1, 0.19, 0.29, 0.19, 0.12, 0.16, 0.06, 0.09, 0.27, 0.37, 0.22, 0.27, 0.7, 0.11], "dc23"=[-0.01, -0.55, -0.07, -0.18, 0.12, -0.7, -0.68, -0.21, -0.24, -0.07, -0.04, 0.3, -0.13, 0.09, 0.01, -0.42, -0.5, -0.17, -0.13, -0.16, -0.03, -0.18, -0.35, 0.02, 0.04, -0.15, -0.08, -0.06, -0.31, -0.2, -0.34, -0.35, -0.98, -0.26], "dc13"=[0.0, 0.24, -1.06, 0.06, -0.32, 0.25, -0.02, 0.16, 0.1, -0.01, -0.15, -0.97, -0.54, -0.75, -0.56, -1.24, 0.07, -0.08, -0.05, -0.06, -0.15, -0.21, -0.16, -0.41, -0.31, -0.19, -0.02, -0.13, -0.12, -0.4, -0.11, -0.09, -0.13, 0.03], "dc12"=[0.0, -0.91, -0.01, -0.18, -0.46, -0.64, -0.07, -1.45, -0.42, -0.02, -0.05, -0.71, -0.78, -0.24, -0.12, 0.29, -0.21, -0.89, -0.04, -0.29, -0.47, 0.01, -0.34, -0.21, -0.36, -0.01, -1.38, -0.07, -0.46, -0.37, -0.01, -0.27, -0.04, -0.18], "dc44"=[0.1, 0.08, 0.02, 0.13, 0.14, 0.0, 0.27, 0.0, 0.22, 0.0, 0.21, 0.0, 0.0, 0.01, 0.11, 0.0, 0.42, 0.0, 0.25, 0.29, 0.0, 0.29, 0.0, 0.09, 0.16, 0.24, 0.0, 0.3, 0.0, 0.0, 0.46, 0.0, 0.0, 0.47], "dc55"=[0.06, 0.01, 0.12, 0.13, 0.11, 0.0, 0.02, 0.0, 0.13, 0.0, 0.17, 0.0, 0.0, 0.33, 0.29, 0.0, 0.01, 0.0, 0.21, 0.16, 0.0, 0.21, 0.0, 0.4, 0.35, 0.3, 0.0, 0.23, 0.0, 0.0, 0.1, 0.0, 0.0, 0.11], "dc66"=[0.82, 0.0, 0.01, 0.5, 0.31, 0.17, 0.02, 0.0, 0.23, 0.92, 0.44, 0.12, 0.01, 0.01, 0.11, 0.01, 0.01, 0.23, 0.34, 0.16, 0.58, 0.17, 0.4, 0.06, 0.04, 0.15, 0.04, 0.26, 0.39, 0.36, 0.01, 0.51, 0.18, 0.07], "all moduli"=["c11", "c22", "c33", "c23", "c13", "c12", "c44", "c55", "c66"], "c33"=0.85415, "c23"=0.90617, "c13"=0.95768, "c12"=1.60744, "c44"=0.45912, "c55"=0.45304, "c66"=0.74548, "d1"=0.09611, "d2"=0.11831, "d3"=0.02141, "dL11"=[0.008042331146684635, -0.8730462686535754, 1.048370328442947, -0.1816165745228517, 0.01125988400118176, -0.6850658839094866, -0.02818303126249565, -1.1605413955282224, -0.3942834596821436, -0.0023077723987954516, 0.11888670177662322, 0.4126774453638666, -0.03370680552622996, 0.6076508918025406, 0.4928202278483594, 1.3242568488254176, -0.2212687232811257, -0.5410029192407099, 0.02755377978914764, -0.14203417026277648, -0.19497344643867404, 0.2303603238799098, -0.09552844880631507, 0.2934404701066909, 0.0871373951686361, 0.17979856460100654, -0.9393424167452952, 0.09245193593777386, -0.2219677192526727, 0.07392001224921144, 0.10741758428084484, -0.11559940442392723, 0.07580776666925547, -0.16553191222948244], "dL12"=[0.0, 0.24, -1.06, 0.06, -0.32, 0.25, -0.02, 0.16, 0.1, -0.01, -0.15, -0.97, -0.54, -0.75, -0.56, -1.24, 0.07, -0.08, -0.05, -0.06, -0.15, -0.21, -0.16, -0.41, -0.31, -0.19, -0.02, -0.13, -0.12, -0.4, -0.11, -0.09, -0.13, 0.03], "dL22"=[0.01, 0.15, 0.56, 0.06, 0.1, 0.23, 0.34, 0.02, 0.07, 0.04, 0.09, 0.35, 0.36, 0.32, 0.26, 0.9, 0.2, 0.14, 0.08, 0.11, 0.1, 0.19, 0.29, 0.19, 0.12, 0.16, 0.06, 0.09, 0.27, 0.37, 0.22, 0.27, 0.7, 0.11], "dL33"=[0.82, 0.0, 0.01, 0.5, 0.31, 0.17, 0.02, 0.0, 0.23, 0.92, 0.44, 0.12, 0.01, 0.01, 0.11, 0.01, 0.01, 0.23, 0.34, 0.16, 0.58, 0.17, 0.4, 0.06, 0.04, 0.15, 0.04, 0.26, 0.39, 0.36, 0.01, 0.51, 0.18, 0.07], "dL44"=[0.001957668853315366, 0.37304626865357543, 0.2616296715570529, 0.07161657452285171, 0.2987401159988182, 0.2450658839094865, 0.038183031262495656, 0.6505413955282222, 0.17428345968214365, 0.012307772398795448, 0.061113298223376786, 0.5573225546361333, 0.49370680552623, 0.30234910819745925, 0.19717977215164073, 0.1357431511745822, 0.08126872328112572, 0.44100291924070995, 0.03244622021085236, 0.15203417026277652, 0.2549734464386741, 0.0496396761200902, 0.19552844880631504, 0.20655952989330914, 0.25286260483136386, 0.05020143539899344, 0.6593424167452954, 0.06754806406222615, 0.2419677192526726, 0.25607998775078855, 0.03258241571915516, 0.14559940442392721, 0.044192233330744554, 0.07553191222948244], "dL55"=[0.1, 0.08, 0.02, 0.13, 0.14, 0.0, 0.27, 0.0, 0.22, 0.0, 0.21, 0.0, 0.0, 0.01, 0.11, 0.0, 0.42, 0.0, 0.25, 0.29, 0.0, 0.29, 0.0, 0.09, 0.16, 0.24, 0.0, 0.3, 0.0, 0.0, 0.46, 0.0, 0.0, 0.47], "L11"=2.124615, "L12"=0.95768, "L22"=0.85415, "L33"=0.74548, "L44"=0.5171749999999999, "L55"=0.45912, "# of free elastic constants"=9, "det12"=[8.042331146684635e-05, -0.18855694029803632, -0.5365126160719498, -0.014496994471371101, -0.10127401159988184, -0.22006515329918194, -0.009982230629248521, -0.04881082791056445, -0.03759984217775006, -0.00019231089595181806, -0.011800196840103909, -0.7964628941226467, -0.3037344499894428, -0.368051714623187, -0.1854667407594266, -0.3457688360571243, -0.04915374465622514, -0.08214040869369939, -0.00029569761686818906, -0.019223758728905412, -0.0419973446438674, -0.0003315384628171311, -0.053303250153831375, -0.1123463106797287, -0.08564351257976367, -0.007332229663838952, -0.05676054500471771, -0.008579325765600354, -0.07433128419822163, -0.13264959546779181, 0.011531868541785867, -0.03931183919446035, 0.03616543666847882, -0.01910851034524307]}
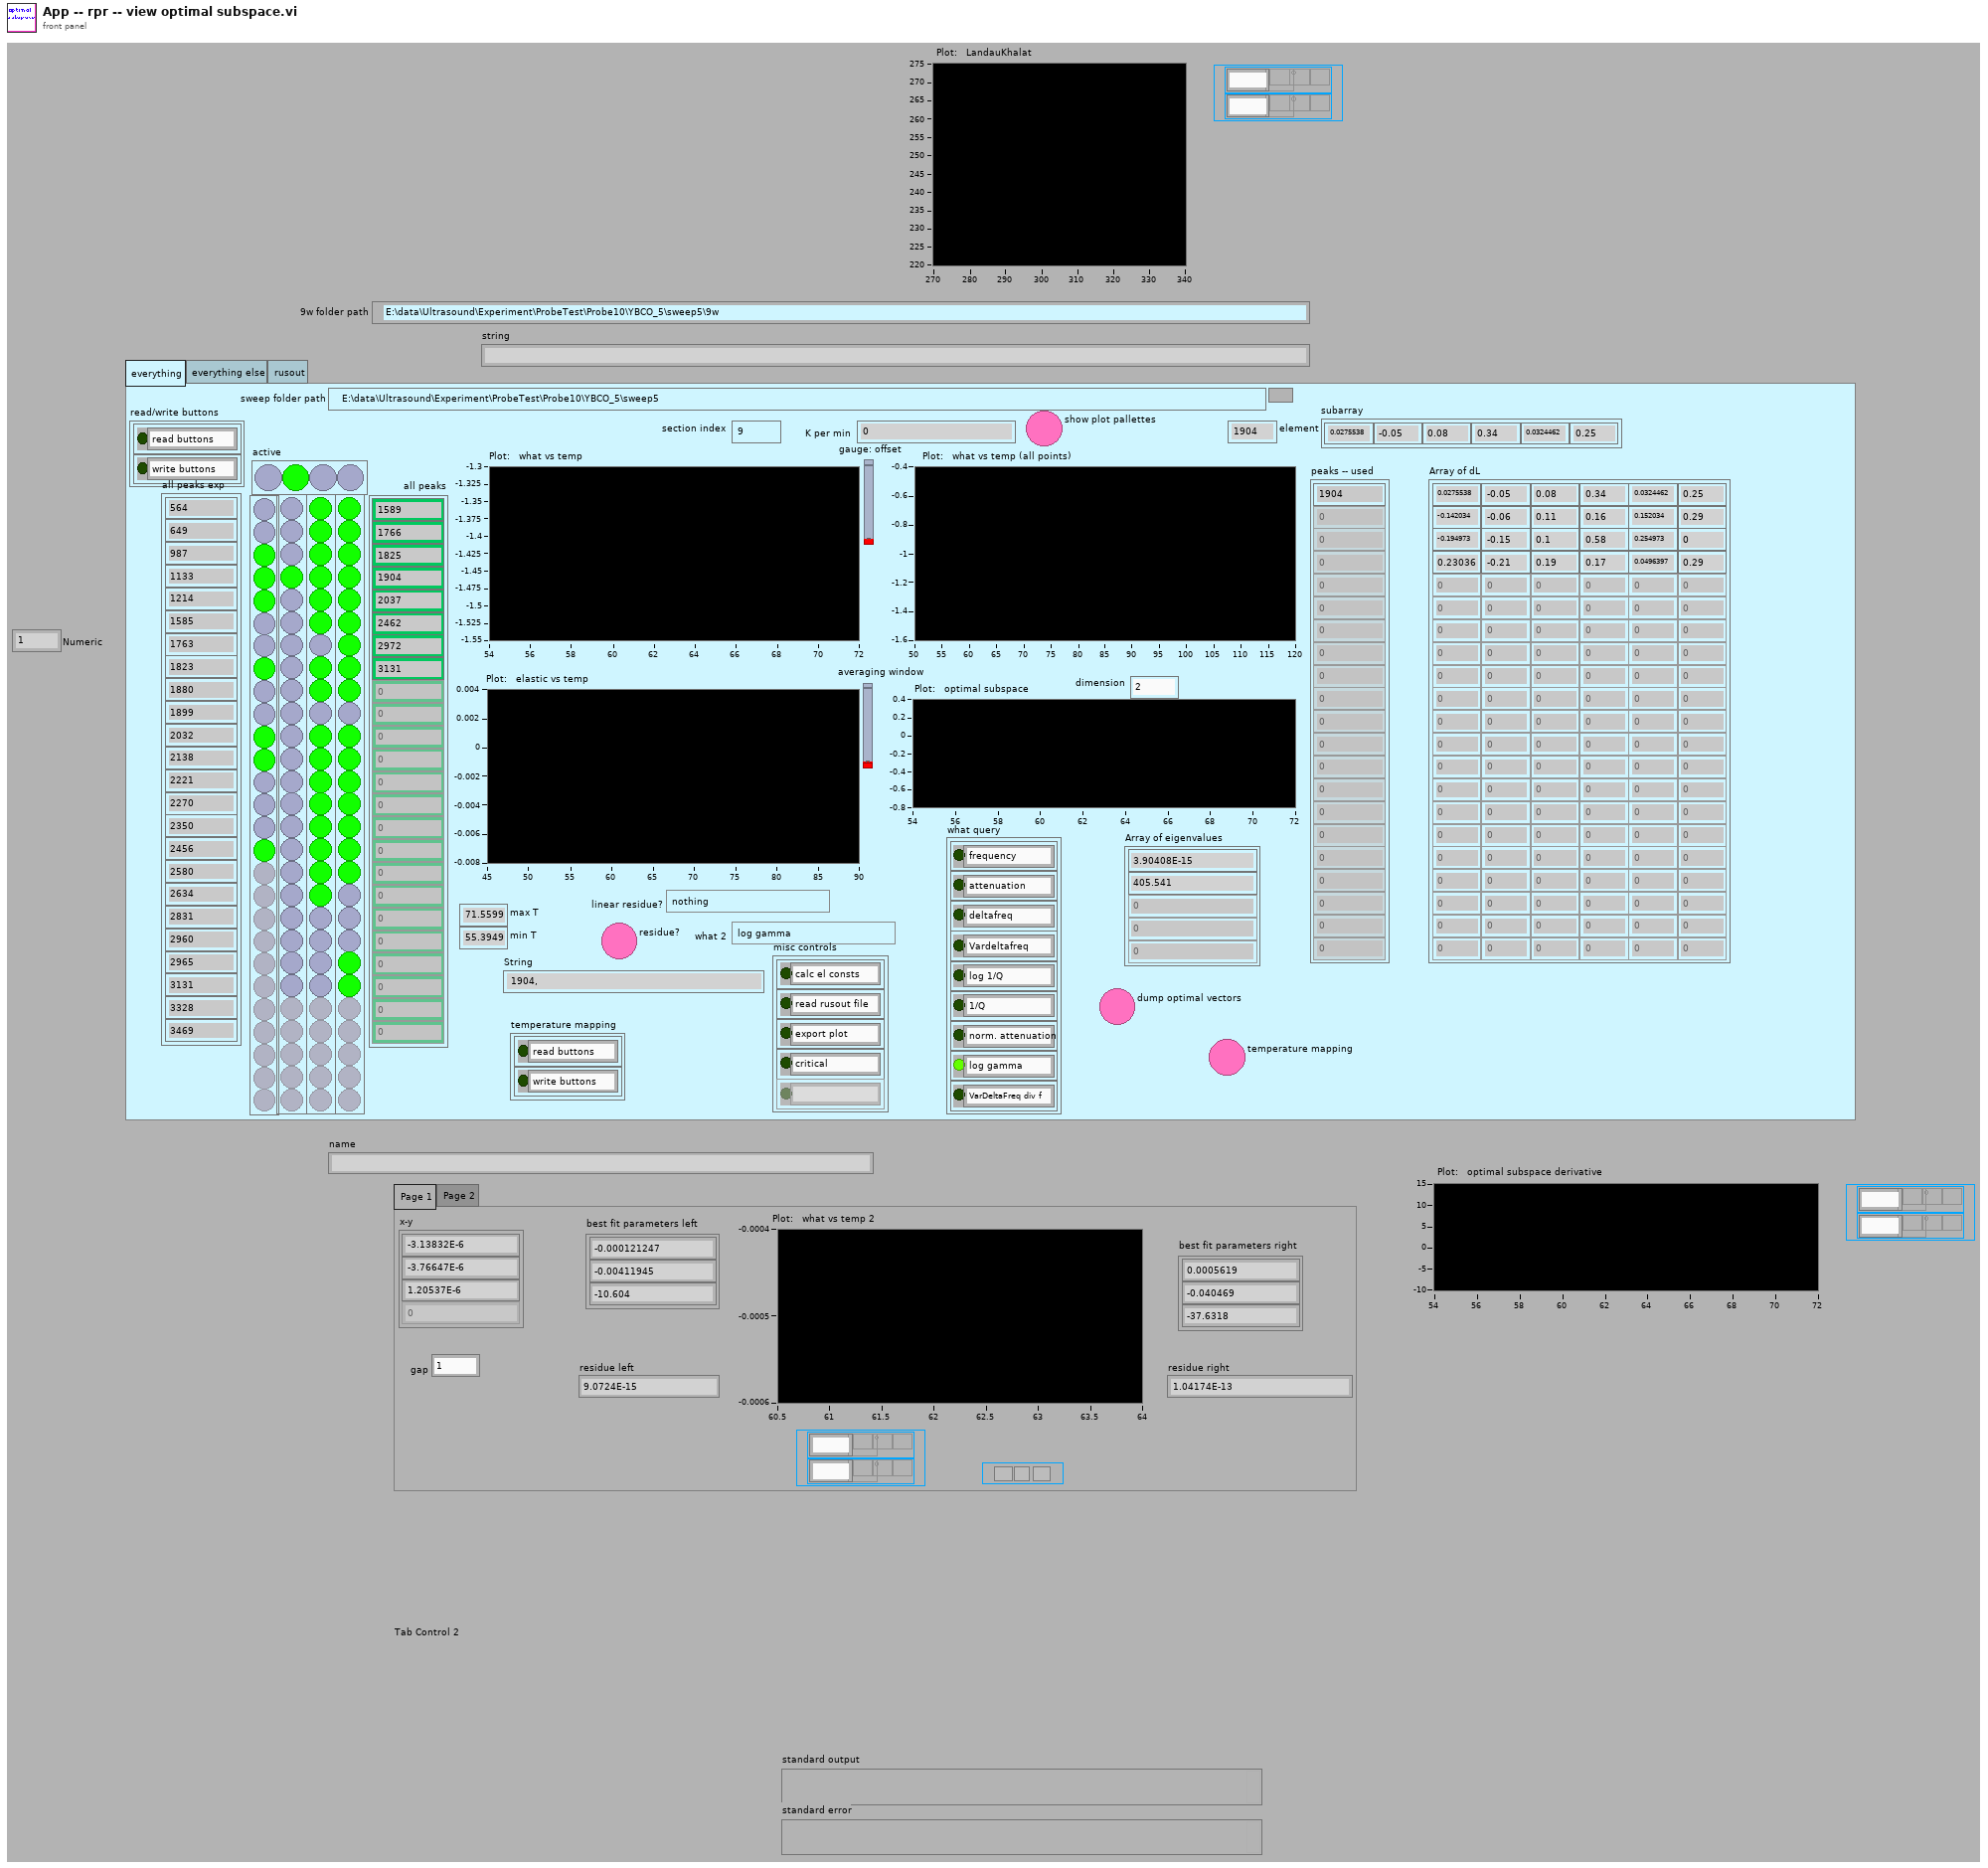
[diagram p1: front panel]
types:
  T1 = enum32{"everything", "everything else", "rusout"}
  T2 = typedef "query.ctl" = cluster{"Boolean":bool, "String":string}
  T3 = enum16{"frequency", "attenuation", "deltafreq", "Vardeltafreq", "log 1/Q", "1/Q", "norm. attenuation", "log gamma", "VarDeltaFreq div f"}
  T4 = typedef "cursor winow.ctl" = cluster{"left":dbl, "right ":dbl, "center":dbl, "window":dbl, "cursors":i32[], "relative":i32, "absolute":i32, "fixed vertical offset":dbl, "vertical offset":dbl, "skew":dbl, "default window frac":dbl, "kind":enum16{"symmetric", "skewed", "fancy"}, "skew.left":dbl, "skew.right":dbl, "Plot ref":refnum<vi>, "wing order":enum16{"forw", "back"}}
  T5 = typedef "link -- rusout - tetragonal.ctl" = cluster{"freqs Exp":dbl[], "symmetry":i32[], "dc11":dbl[], "freqs Fit":dbl[], "header":string, "bulk modulus":dbl, "c11":dbl, "c22":dbl, "free moduli":string[], "# of polynomials":i32, "mass, g":dbl, "density, g/cm3":dbl, "dc22":dbl[], "dc33":dbl[], "dc23":dbl[], "dc13":dbl[], "dc12":dbl[], "dc44":dbl[], "dc55":dbl[], "dc66":dbl[], "all moduli":string[], "c33":dbl, "c23":dbl, "c13":dbl, "c12":dbl, "c44":dbl, "c55":dbl, "c66":dbl, "d1":dbl, "d2":dbl, "d3":dbl, "dL11":dbl[], "dL12":dbl[], "dL22":dbl[], "dL33":dbl[], "dL44":dbl[], "dL55":dbl[], "L11":dbl, "L12":dbl, "L22":dbl, "L33":dbl, "L44":dbl, "L55":dbl, "# of free elastic constants":i32, "det12":dbl[]}
  T6 = typedef "tfolder.ctl" = cluster{"tfolder path":path, "9folder path":path, "tfolder  -  file array":T7[], "from index array":i32[], "timestamp array":dbl[]}
  T7 = typedef "tfolder -- monotonic segment.ctl" = cluster{"timestamp from":dbl, "timestamp to":dbl, " index  from":i32, "index to":i32, "active":bool}
  T8 = typedef "cursor window action.ctl" = enum16{"balance", "h. offset change", "cursor moves", "change center", "change window", "init", "check", "reset", "set y to middle", "idle", "-write all Y", "-write left.X", "-write center.X", "-write right.X", "-write all X", "-change center", "-change window", "-change skew", "-read cursor 2", "-read cursor 1", "-read cursor 0", "-read all cursors", "-reset", "-read plot scale", "-set y to middle", "-Q: center.Y is visible", "-Q: window is visible", "-parse center.Y", "-right left from center", "-left move", "-right move", "-set center.Y", "-empty", "-set cursors to default", "-check", "-write center.Y", "-copy cursor 1", "-copy cursor 0", "-copy cursor 2", "move right", "move left", "shrink", "broaden", "skew up", "skew down", "-write plot scale", "zoom X", "change cen&win", "zoom to all data"}
  T9 = cluster{"left":dbl, "right ":dbl, "center":dbl, "window":dbl, "cursors":i32[], "relative":i32, "absolute":i32, "fixed vertical offset":dbl, "vertical offset":dbl, "skew":dbl, "default window frac":dbl, "kind":enum16{"symmetric", "skewed", "fancy"}, "skew.left":dbl, "skew.right":dbl, "Plot ref":refnum<vi>, "wing order":enum16{"forw", "back"}}
  T10 = cluster{"temperature points OUT":dbl[], "delta freq points OUT":dbl[]}[]
  T11 = cluster{"temperature points OUT":dbl[], "Array":dbl[]}
  T12 = cluster{"temperature points OUT":dbl[], "what points out":dbl[]}
  T13 = cluster{"temperature points OUT":dbl[], "what points out":dbl[]}[]
  T14 = typedef "NI_Matrix.lvlib/RealMatrix.ctl" = dbl[][]
  T15 = cluster{"temperature points OUT":dbl[], "Real 2D Array":dbl[]}
  T16 = typedef "LVPoint32TypeDef.ctl" = cluster{"Horizontal":i32, "Vertical":i32}
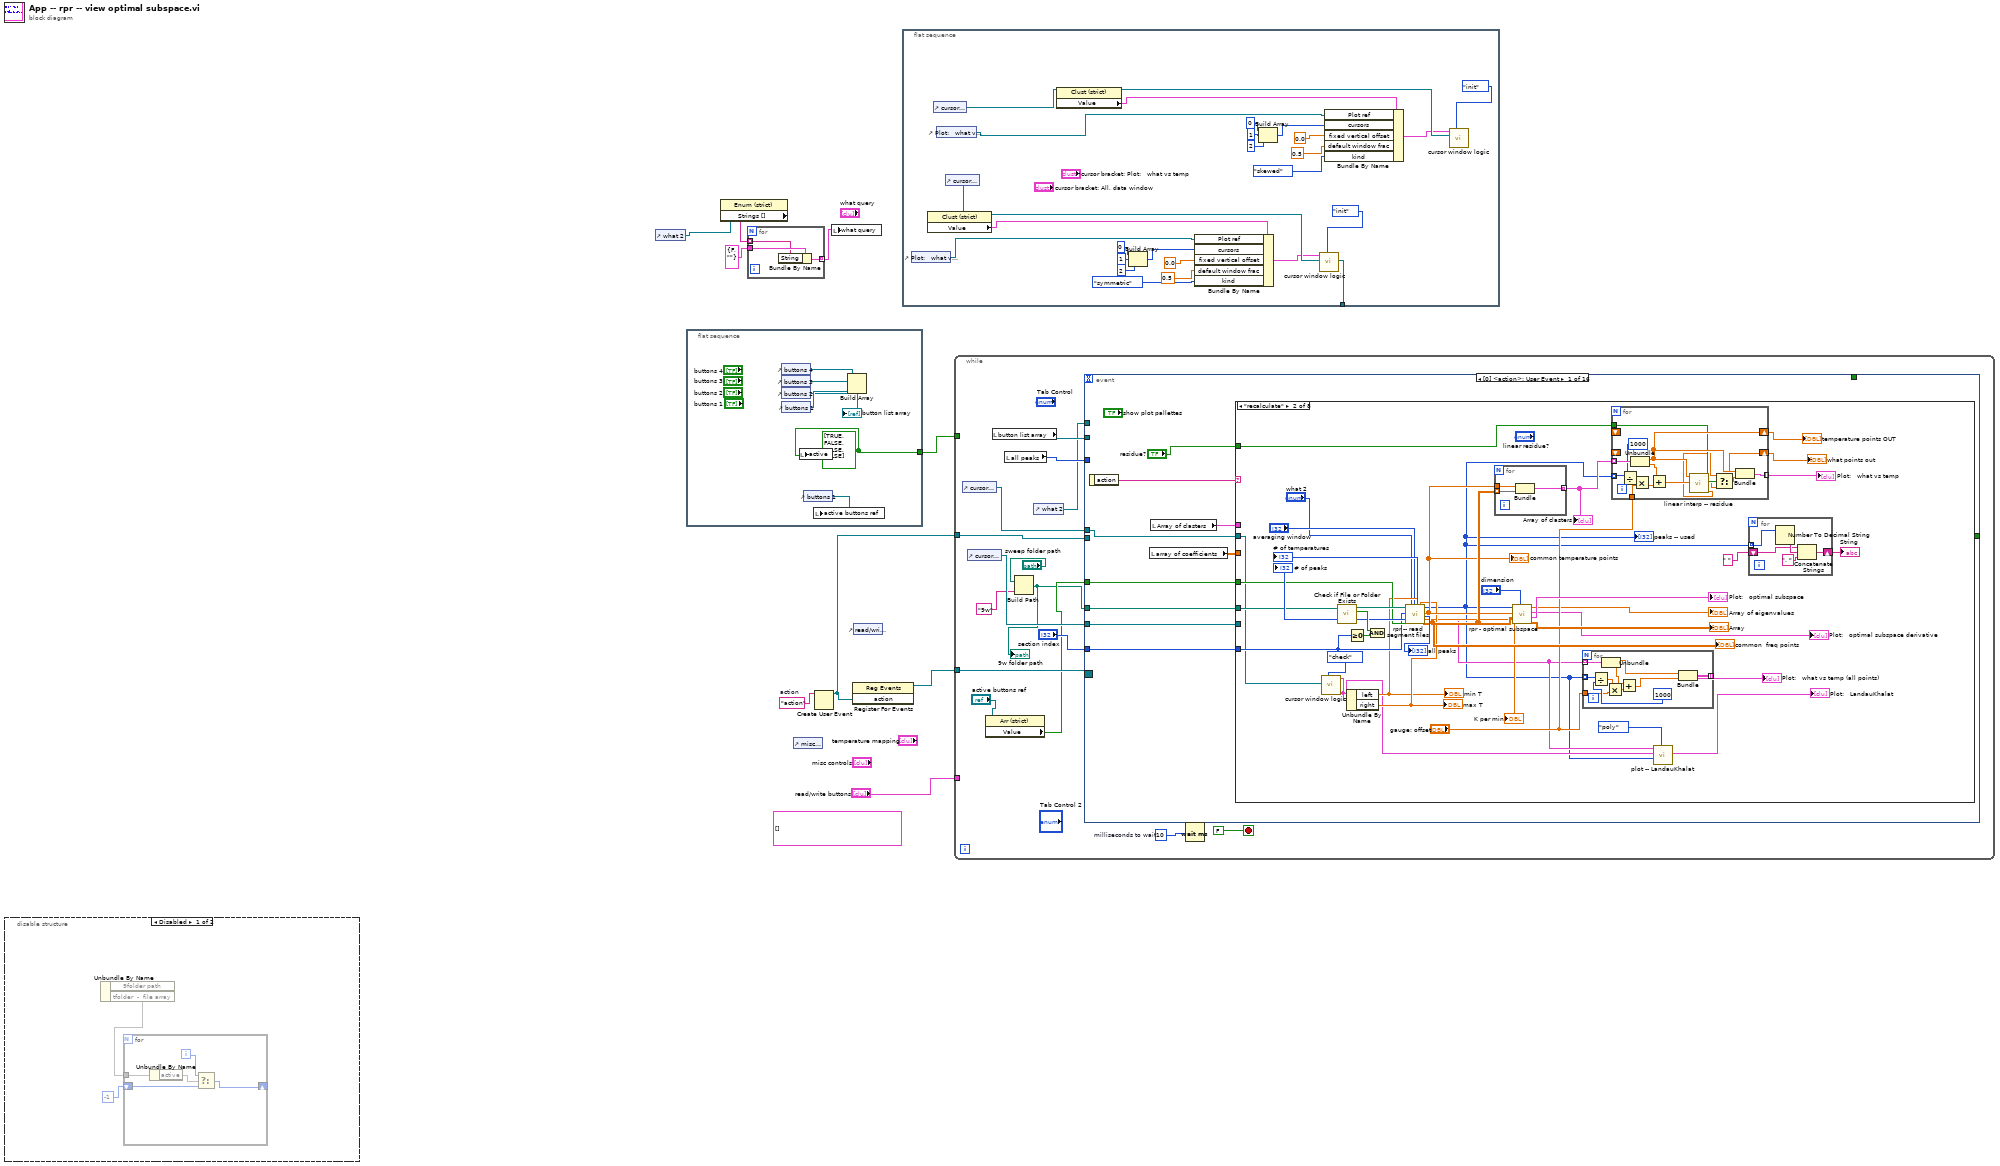
[diagram p0: block diagram]
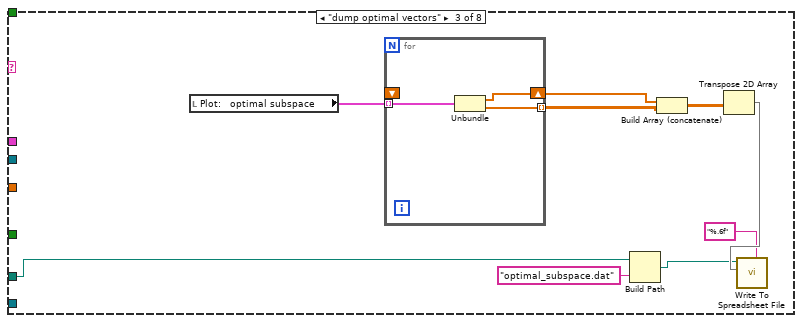
[diagram p3: hidden frame]
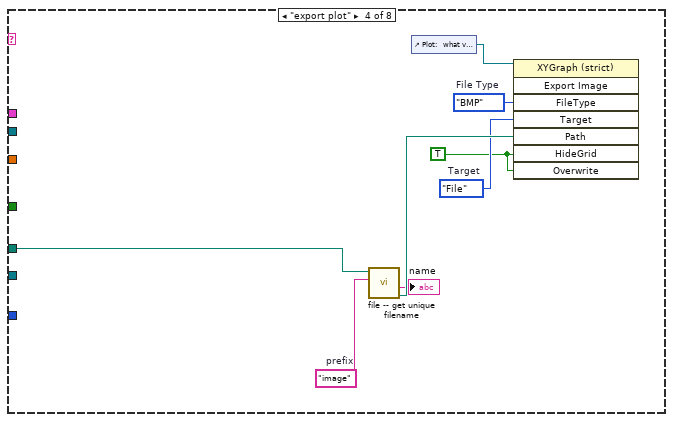
[diagram p4: hidden frame]
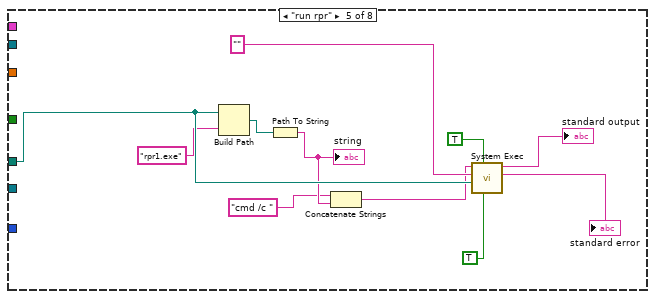
[diagram p5: hidden frame]
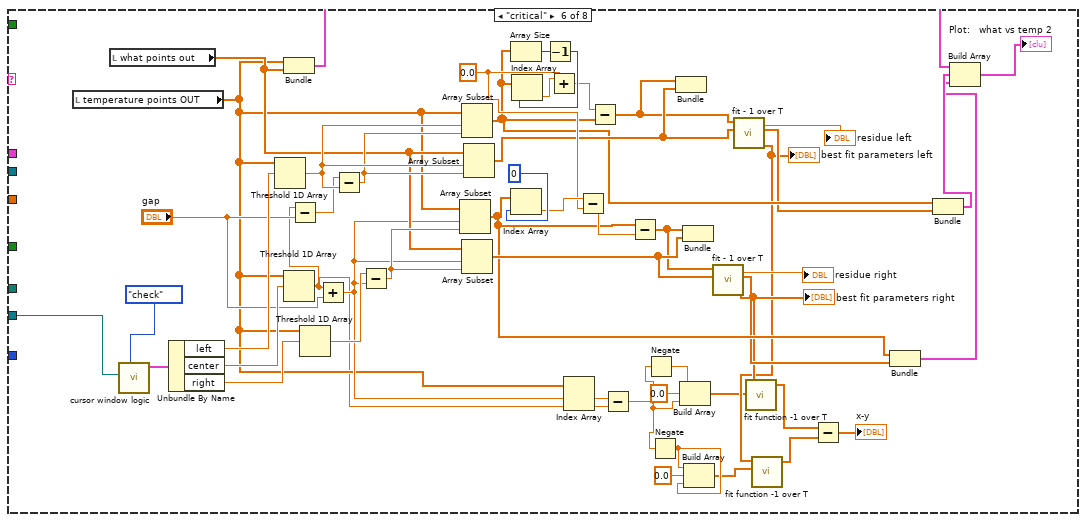
[diagram p6: hidden frame]
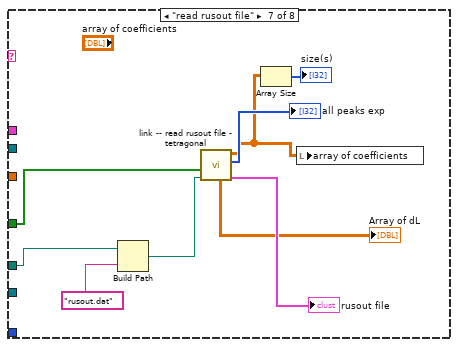
[diagram p7: hidden frame]
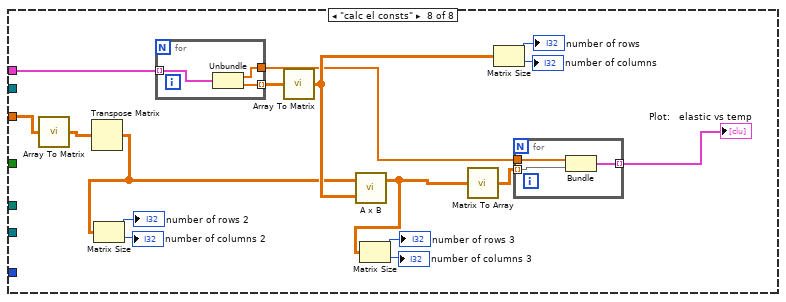
[diagram p8: hidden frame]
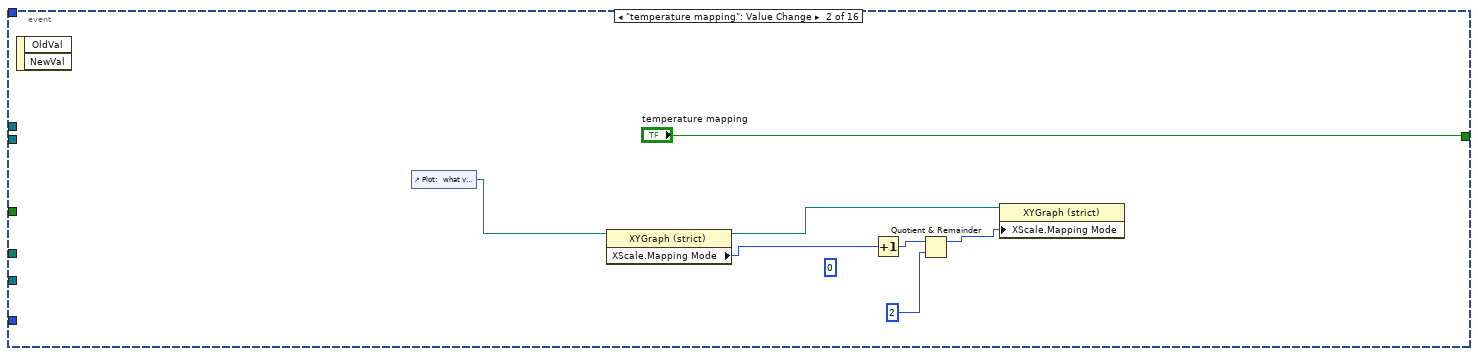
[diagram p9: hidden frame]
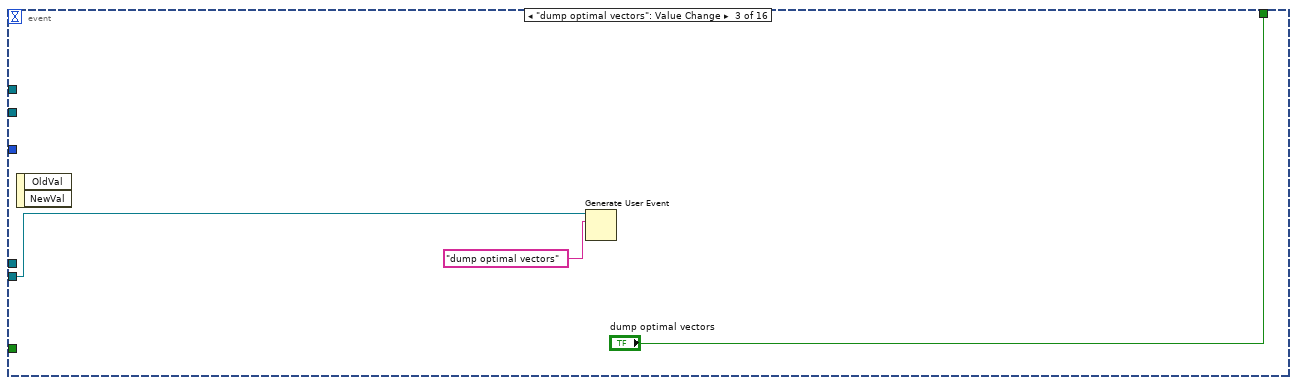
[diagram p10: hidden frame]
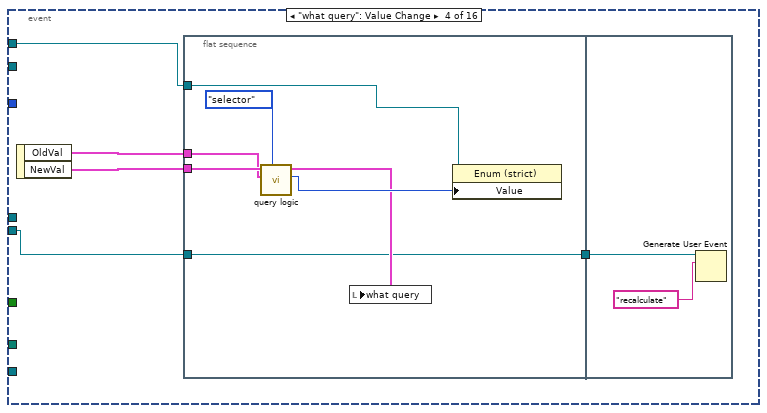
[diagram p11: hidden frame]
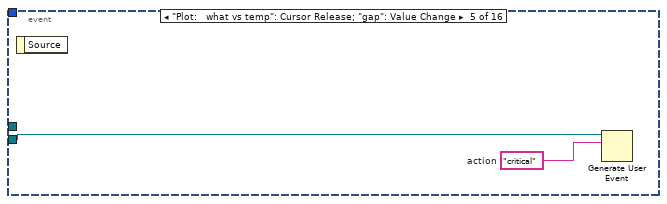
[diagram p12: hidden frame]
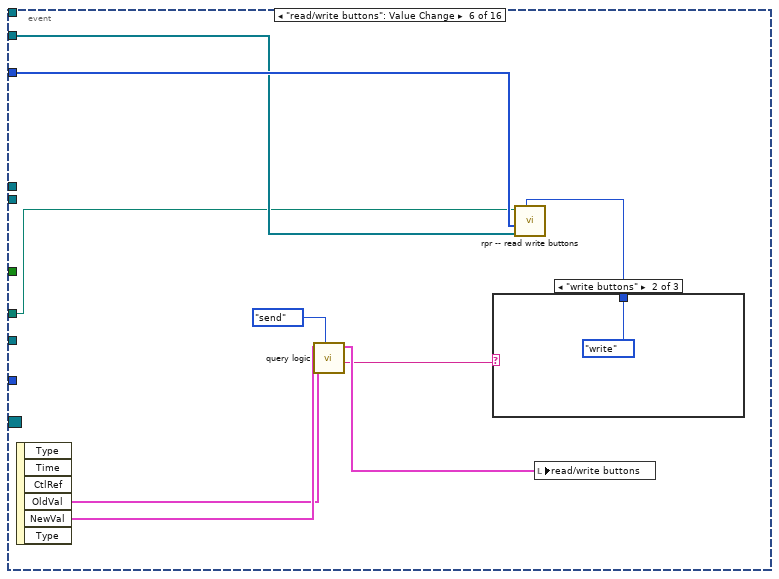
[diagram p13: hidden frame]
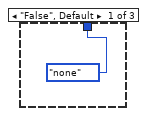
[diagram p14: hidden frame]
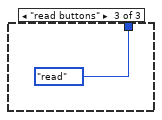
[diagram p15: hidden frame]
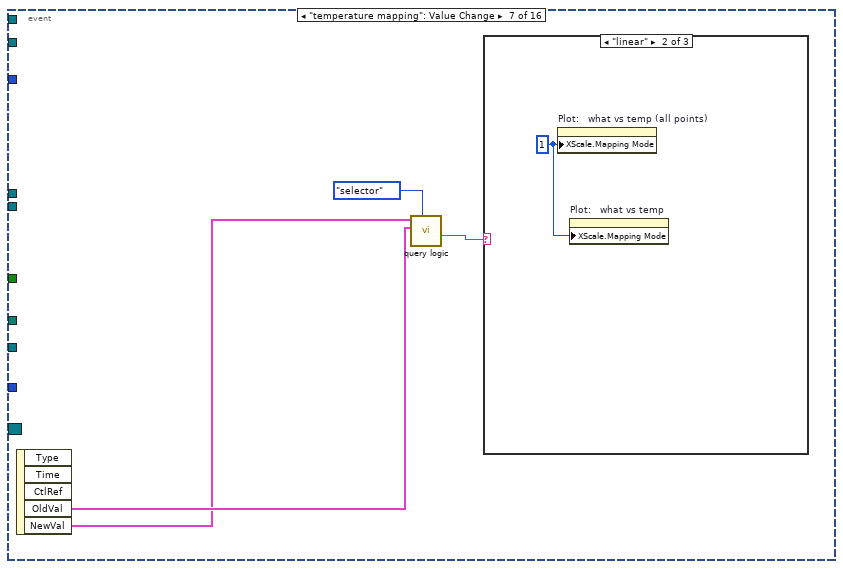
[diagram p16: hidden frame]
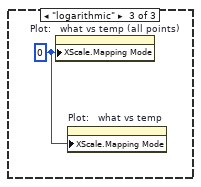
[diagram p18: hidden frame]
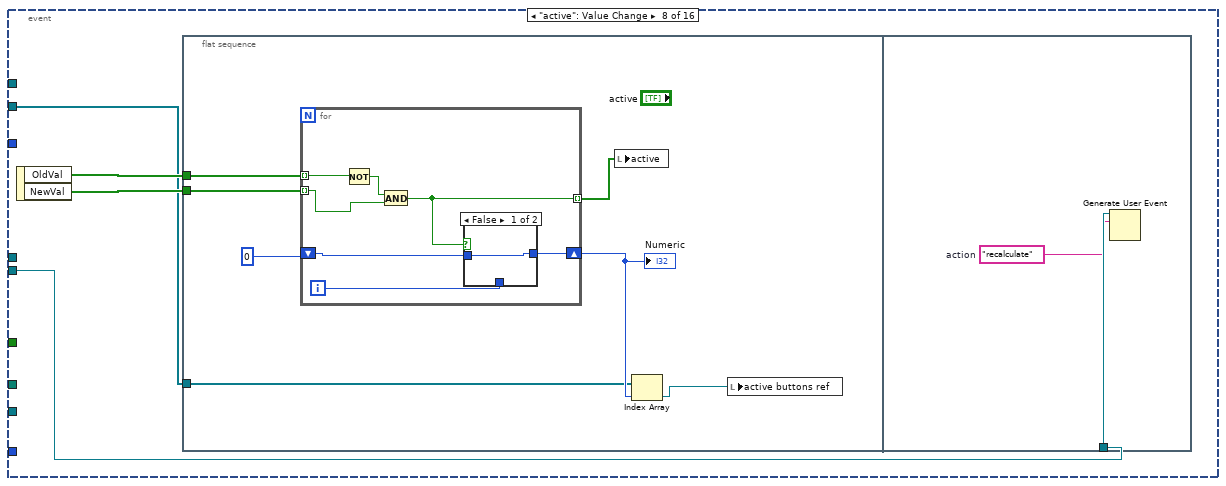
[diagram p19: hidden frame]
diagram:
  (unwired) T2[] [] ("read/write buttons")
  w8 = "action"  # action
  n1 = disable-structure shown="Disabled" {
    frame Disabled {
      n2 = Unbundle By Name() -> (w14:T6, "9folder path"=w13, "tfolder  -  file array"=w12)
      n3 = for {
        tunnel: w12 -> [w19]
        shift-right: [w15] -> w10
        shift-left: -1 -> [w16]
        i -> [w17]
        n4 = Unbundle By Name(w19) -> ("active"=w18)
        n5 = Select(t=w17, s=w18, f=w16) -> (s? t:f=w15:i32)
      }
    }
    frame Enabled {
    }
  }
  n6 = control-ref of="what 2"() -> (w1:refnum<vi>)
  n7 = flat-sequence {
    tunnel: [w25] -> w6
    frame #0 {
      w25 = bool[] [TRUE, FALSE, FALSE, FALSE] ("active")
      n8 = control-ref of="buttons 4"() -> (w21:refnum<vi>)
      n9 = control-ref of="buttons 3"() -> (w22:refnum<vi>)
      n10 = control-ref of="buttons 2"() -> (w23:refnum<vi>)
      n11 = control-ref of="buttons 1"() -> (w24:refnum<vi>)
      n12 = local write "active"(w25) -> ()
      n13 = control-ref of="buttons 1"() -> (w26:refnum<vi>)
      n14 = local write "active buttons ref"(w26) -> ()
      n15 = Build Array(w21, w22, w23, w24) -> (→"button list array":refnum<vi>[])
    }
  }
  n16 = property class="Enum (strict)"(reference=w1) -> ("Strings []"=w2:string[])  [unwired: 1 in, 2 out]
  n17 = for {
    tunnel: w2 -> [w28] mode=indexing
    tunnel: T2 {"Boolean"=FALSE, "String"=""} ("query") -> [w29]
    tunnel: [w27] -> w4 mode=indexing
    n18 = Bundle By Name(cluster=w29, "String"=w28) -> (w27:T2)
  }
  n19 = control-ref of="misc controls"() -> ()  [unwired: 1 out]
  n20 = Create User Event(user event datatype=w8) -> (user event=w7:refnum<user-event>)  [unwired: 1 in, 1 out]
  n21 = local write "what query"(w4) -> ()
  n22 = register-events(w7) -> (reference out=w9:refnum<event-registration>)  [unwired: 2 in, 1 out]
  n23 = control-ref of="read/write buttons"() -> ()  [unwired: 1 out]
  n24 = flat-sequence {
    tunnel: [w45] -> _
    frame #0 {
      n25 = control-ref of="Plot:   what vs temp (all points)"() -> (w44:refnum<vi>)
      n26 = control-ref of="cursor bracket: Plot:   what vs temp"() -> (w30:refnum<vi>)
      n27 = control-ref of="Plot:   what vs temp"() -> (w31:refnum<vi>)
      n28 = control-ref of="cursor bracket: All, data window"() -> (w48:refnum<vi>)
      n29 = property class="Clust (strict)"(reference=w48) -> (reference out=w49:refnum<vi>, "Value"=w47:T9)  [unwired: 1 in, 1 out]
      n30 = property class="Clust (strict)"(reference=w30) -> (reference out=w35:refnum<vi>, "Value"=w34:T9)  [unwired: 1 in, 1 out]
      n31 = Build Array(0, 1, 2) -> (w56:i32[])
      n32 = Bundle By Name(cluster=w47, "Plot ref"=w44, "cursors"=w56, "fixed vertical offset"=0.0, "default window frac"=0.5 ("fixed vertical offset"), "kind"=enum16{"symmetric", "skewed", "fancy"}."symmetric") -> (w46:T9)
      n33 = Build Array(0, 1, 2) -> (w42:i32[])
      n34 = call "cursor window logic.vi"("cursor window action"=cursor_window_action."init", 10:"cursor bracket in"=w49, 11:"cursor bracket in"=w46) -> ("reference out"=w45:refnum<vi>)  [unwired: 7 in, 1 out]
      n35 = Bundle By Name(cluster=w34, "Plot ref"=w31, "cursors"=w42, "fixed vertical offset"=0.0, "default window frac"=0.5 ("fixed vertical offset"), "kind"=enum16{"symmetric", "skewed", "fancy"}."skewed") -> (w33:T9)
      n36 = call "cursor window logic.vi"("cursor window action"=cursor_window_action."init", 10:"cursor bracket in"=w35, 11:"cursor bracket in"=w33) -> ()  [unwired: 7 in, 2 out]
    }
  }
  n37 = while {
    tunnel: w9 -> [w69]
    tunnel: w7 -> [w68]
    tunnel: w6 -> [_]
    tunnel: "read/write buttons" -> [_]
    stop <- FALSE stop-if-true
    w71 = u32 10  # milliseconds to wait
    n38 = control-ref of="cursor bracket: All, data window"() -> (w66:refnum<vi>)
    n39 = control-ref of="cursor bracket: Plot:   what vs temp"() -> (w65:refnum<vi>)
    n40 = property class="Arr (strict)"(reference="active buttons ref") -> ("Value"=w63:bool[])  [unwired: 1 in, 2 out]
    n41 = local read "button list array"() -> (w61:refnum<vi>[])
    n42 = local read "all peaks"() -> (w62:i32[])
    n43 = Build Path(base path="sweep folder path", name or relative path="9w" ("action")) -> (appended path=w58:path)
    "9w folder path" <- w58
    n44 = control-ref of="what 2"() -> (w57:refnum<vi>)
    n45 = event shown="[0] <action>: User Event" {
      selector: w69 -> [_ _ _ _ _ _ _ _ _ _ _ _ _ _ _ _]
      dyn-events: _ -> [_ _ _ _ _ _ _ _ _ _ _ _ _ _ _ _]
      timeout: _ -> [_ _ _ _ _ _ _ _ _ _ _ _ _ _ _ _]
      tunnel: w68 -> [_ _ w271 w276 w288 _ _ w309 _ _ _ _ w373 w375 w376 _]
      tunnel: w58 -> [w80 _ _ _ _ w296 _ _ _ _ _ _ _ _ _ _]
      tunnel: w63 -> [w79 _ _ _ _ _ _ _ _ _ w343 _ _ _ _ _]
      tunnel: "section index" -> [w78 _ _ _ _ _ _ _ _ _ _ _ _ _ _ _]
      tunnel: w66 -> [w74 _ _ _ _ _ _ _ w331 _ _ w366 _ _ _ _]
      tunnel: w65 -> [w73 _ _ _ _ _ _ _ _ w334 _ _ _ _ _ _]
      tunnel: w62 -> [_ _ _ _ _ w298 _ _ _ _ _ _ _ _ _ _]
      tunnel: w61 -> [_ _ _ _ _ w297 _ w308 _ _ _ _ _ _ _ _]
      tunnel: w57 -> [_ _ _ w274 _ _ _ _ _ _ _ _ _ _ _ _]
      tunnel: [_ _ "dump optimal vectors" _ _ _ _ _ _ _ _ _ _ _ _ _] -> _
      tunnel: [_ "temperature mapping" _ _ _ _ _ _ _ _ _ _ _ _ _ _] -> _
      event User Event {
        n46 = event-data() -> ("action"=w77:string)  [unwired: 1 in]
        n47 = local read "array of coefficients"() -> (w75:dbl[][])
        n48 = local read "Array of clasters"() -> (w76:cluster{"temperature points OUT":dbl[], dbl[]}[])
        n49 = case shown="\"recalculate\"" w77 {
          tunnel: w80 -> [_ w107 w157 w163 w178 _ w241 _]
          tunnel: w79 -> [_ w106 _ _ _ _ w237 _]
          tunnel: w78 -> [_ w105 _ _ _ _ _ _]
          tunnel: w76 -> [_ _ _ _ _ _ _ w257]
          tunnel: w75 -> [_ _ _ _ _ _ _ w253]
          tunnel: w74 -> [_ w96 _ _ _ _ _ _]
          tunnel: w73 -> [_ _ _ _ _ w232 _ _]
          tunnel: "residue?" -> [_ w87 _ _ _ _ _ _]
          frame "False", Default {
          }
          frame "recalculate" {
            n50 = call "cursor window logic.vi"("cursor window action"=cursor_window_action."check", "cursor bracket in"=w96) -> ("cursor window out"=w84:T4)  [unwired: 8 in, 1 out]
            n51 = call <vilib>:"Check if File or Folder Exists.vi"("path"=w107) -> ("file or folder exists?"=w116:bool, "dup path"=w117:path)  [unwired: 8 in, 1 out]
            n52 = Unbundle By Name(w84) -> ("left"=w102:dbl, "right"=w103:dbl)
            "max T" <- w103
            "min T" <- w102
            n53 = Greater Or Equal To 0?(x=w105) -> (x >= 0?=w115:bool)
            n54 = And(x=w116, y=w115) -> ()  [unwired: 1 out]
            n55 = call "rpr -- read segment files.vi"("9w folder path"=w117, "segment index"=w105, "buttons"=w106, "what"="what 2", "averaging window"="averaging window", "min T"=w102, "max T"=w103) -> ("# of peaks"=→"# of peaks":i32, "# of temperatures"=→"# of temperatures":i32, "K per min"=→"K per min":dbl, "peaks"=w83:i32[], "temperature points OUT"=w110:dbl[], "all peaks"=→"all peaks":i32[], "all unfiltered"=w85:T10, "Array"=w111:dbl[][])  [unwired: 5 in]
            "peaks -- used" <- w83
            "common temperature points" <- w110
            "common  freq points" <- w111
            n56 = for {
              tunnel: w111 -> [w148] mode=indexing
              tunnel: w110 -> [w149]
              tunnel: [w147] -> w100 mode=indexing
              n57 = Bundle("temperature points OUT"=w149, "Array"=w148) -> (w147:T11)  [unwired: 1 in]
            }
            "Array of clasters" <- w100
            n58 = call "rpr - optimal subspace.vi"("dimension"="dimension", "Array of peaks IN"=w111, "temperature points"=w110, "peaks"=w83) -> ("Array"=→"Array":dbl[][], "Array of clasters"=→"Plot:   optimal subspace":cluster{"temperature points OUT":dbl[], dbl[]}[], "Array of clasters derivative"=→"Plot:   optimal subspace derivative":cluster{"temperature points OUT":dbl[], dbl[]}[], "Array of eigenvalues"=→"Array of eigenvalues":dbl[])  [unwired: 4 in]
            n59 = for {
              tunnel: w85 -> [w146] mode=indexing
              tunnel: w83 -> [w137] mode=indexing
              tunnel: "gauge: offset" -> [w143]
              tunnel: [w141] -> w101 mode=indexing
              n60 = Divide(x=w137, y=1000) -> (x/y=w144:dbl)
              n61 = Unbundle(w146) -> ("temperature points OUT"=w139:dbl[], "delta freq points OUT"=w138:dbl[])
              n62 = Multiply(x=w144, y=w143) -> (x*y=w142:dbl)
              n63 = Add(x=w138, y=w142) -> (x+y=w140:dbl[])
              n64 = Bundle("temperature points OUT"=w139, w140) -> (w141:cluster{"temperature points OUT":dbl[], dbl[]})  [unwired: 1 in]
            }
            "Plot:   what vs temp (all points)" <- w101
            n65 = for {
              tunnel: w100 -> [w136] mode=indexing
              tunnel: w83 -> [w135] mode=indexing
              tunnel: "gauge: offset" -> [w132]
              tunnel: [w129] -> w99 mode=indexing
              shift-right: [w128] -> w94
              shift-left: _ -> [_]
              shift-right: [w123] -> w93
              shift-left: _ -> [_]
              tunnel: w87 -> [w126]
              n66 = Divide(x=w135, y=1000) -> (x/y=w133:dbl)
              n67 = Unbundle(w136) -> ("temperature points OUT"=w128:dbl[], "Array"=w130:dbl[])
              n68 = Multiply(x=w133, y=w132) -> (x*y=w131:dbl)
              n69 = Add(x=w130, y=w131) -> (x+y=w127:dbl[])
              n70 = call "linear interp -- residue.vi"("what points in"=w127, "temperature points in"=w128) -> ("resudue points out"=w125:dbl[], "what points out"=w124:dbl[])  [unwired: 7 in, 1 out]
              n71 = Select(t=w125, s=w126, f=w124) -> (s? t:f=w123:dbl[])
              n72 = Bundle("temperature points OUT"=w128, "what points out"=w123) -> (w129:T12)  [unwired: 1 in]
            }
            "Plot:   what vs temp" <- w99
            "temperature points OUT" <- w94
            "what points out" <- w93
            n73 = call "plot -- LandauKhalat.vi"("method"=enum16{"max", "parab", "poly"}."poly" ("Enum"), "peaks"=w83, "cursor window out"=w84, "all unfiltered"=w85) -> ("Plot:   LandauKhalat"=→"Plot:   LandauKhalat":cluster{"Array":dbl[], dbl[]}[])  [unwired: 7 in]
            n74 = for {
              tunnel: w83 -> [w122] mode=indexing
              shift-right: [w119] -> w90
              shift-left: " " -> [w118]
              n75 = Number To Decimal String(number=w122) -> (decimal integer string=w121:string)  [unwired: 1 in]
              n76 = Concatenate Strings(w118, w121, ", ") -> (w119:string)
            }
            "String" <- w90
          }
          frame "dump optimal vectors" {
            n77 = local read "Plot:   optimal subspace"() -> (w158:cluster{dbl[], dbl[]}[])
            n78 = for {
              tunnel: w158 -> [w161] mode=indexing
              tunnel: [w160] -> w154 mode=indexing
              shift-right: [w159] -> w155
              shift-left: _ -> [_]
              n79 = Unbundle(w161) -> (w159:dbl[], w160:dbl[])
            }
            n80 = Build Path(base path=w157, name or relative path="optimal_subspace.dat") -> (appended path=w151:path)
            n81 = Build Array (concatenate)(w155, w154) -> (w153:dbl[][])
            n82 = Transpose 2D Array(2D array=w153) -> (transposed array=w152:dbl[][])
            n83 = call-poly <vilib>:"Write To Spreadsheet File.vi"("format (%.3f)"="%.6f", "2D data"=w152, "file path (dialog if empty)"=w151) -> ()  [unwired: 5 in, 1 out]
          }
          frame "export plot" {
            w164 = TRUE
            w165 = enum32{"File", "Clipboard"}."File"  # Target
            w166 = enum32{"BMP", "EPS", "EMF", "PICT"}."BMP"  # File Type
            w168 = "image"  # prefix
            n84 = call "file -- get unique filename.vi"("prefix"=w168, "9w folder path"=w163) -> ("appended path"=w167:path, "name"=→"name":string)  [unwired: 8 in]
            n85 = control-ref of="Plot:   what vs temp (all points)"() -> (w169:refnum<vi>)
            n86 = invoke class="XYGraph (strict)" method="Export Image"(reference=w169, "FileType"=w166, "Target"=w165, "Path"=w167, "HideGrid"=w164, "Overwrite"=w164) -> ()  [unwired: 2 in, 8 out]
          }
          frame "run rpr" {
            n87 = Build Path(base path=w178, name or relative path="rpr1.exe") -> (appended path=w179:path)
            n88 = Path To String(path=w179) -> (string=w173:string)
            "string" <- w173
            n89 = Concatenate Strings("cmd /c ", w173) -> (w171:string)
            n90 = call <vilib>:"System Exec.vi"("run minimized? (F)"=TRUE, "wait until completion? (T)"=TRUE, "working directory"=w178, "standard input"="", "command line"=w171) -> ("standard error"=→"standard error":string, "standard output"=→"standard output":string)  [unwired: 3 in, 2 out]
          }
          frame "critical" {
            w216 = 0.0 ("y")
            n91 = local read "temperature points OUT"() -> (w195:dbl[])
            n92 = local read "what points out"() -> (w211:dbl[])
            n93 = call "cursor window logic.vi"("cursor window action"=cursor_window_action."check", "cursor bracket in"=w232) -> ("cursor window out"=w231:T4)  [unwired: 8 in, 1 out]
            n94 = Unbundle By Name(w231) -> ("left"=w229:dbl, "center"=w228:dbl, "right"=w227:dbl)
            n95 = Threshold 1D Array(2:w229, 3:w195) -> (0:w226:dbl)  [unwired: 1 in]
            n96 = Bundle("temperature points OUT"=w195, "what points out"=w211) -> (w210:T12)  [unwired: 1 in]
            n97 = Threshold 1D Array(2:w228, 3:w195) -> (0:w194:dbl)  [unwired: 1 in]
            n98 = Subtract(x=w194, y="gap") -> (x-y=w201:dbl)
            n99 = Threshold 1D Array(2:w227, 3:w195) -> (0:w223:dbl)  [unwired: 1 in]
            n100 = Add(x=w194, y="gap") -> (x+y=w196:dbl)
            n101 = Subtract(x=w201, y=w226) -> (x-y=w225:dbl)
            n102 = Subtract(x=w223, y=w196) -> (x-y=w224:dbl)
            n103 = Array Subset(array=w195, index=w196, length=w224) -> (w209:dbl[])
            n104 = Array Subset(array=w195, index=w226, length=w225) -> (w208:dbl[])
            n105 = Array Subset(array=w211, index=w196, length=w224) -> (w213:dbl[])
            n106 = Array Subset(array=w211, index=w226, length=w225) -> (w214:dbl[])
            n107 = Array Size(array=w208) -> (size(s)=w222:i32)
            n108 = Index Array(array=w209, index=0) -> (element=w217:dbl)
            n109 = Decrement(x=w222) -> (x-1=w221:i32)
            n110 = Index Array(array=w208, index=w221) -> (element=w220:dbl)
            n111 = Add(x=w220, y=w216) -> (x+y=w219:dbl)
            n112 = Index Array(array=w195, index #1=w196, index #2=w194) -> (element #1=w193:dbl, element #2=w192:dbl)
            n113 = Subtract(x=w217, y=w216) -> (x-y=w215:dbl)
            n114 = Subtract(x=w219, y=w208) -> (x-y=w202:dbl[])
            n115 = Subtract(x=w193, y=w192) -> (x-y=w187:dbl)
            n116 = Subtract(x=w209, y=w215) -> (x-y=w203:dbl[])
            n117 = Negate(x=w187) -> (-x=w191:dbl)
            n118 = Negate(x=w187) -> (-x=w186:dbl)
            n119 = Bundle(w202, w214) -> ()  [unwired: 1 in, 1 out]
            n120 = Build Array(w191, 0.0 ("y"), w187) -> (w189:dbl[])
            n121 = Bundle(w203, w213) -> ()  [unwired: 1 in, 1 out]
            n122 = Build Array(w186, 0.0 ("y"), w186) -> (w185:dbl[])
            n123 = call "fit - 1 over T.vi"("what points"=w213, "temperature points"=w203) -> ("best fit parameters"=w197:dbl[], "what points out"=w205:dbl[], "residue"=→"residue right":dbl)  [unwired: 5 in, 2 out]
            "best fit parameters right" <- w197
            n124 = call "fit - 1 over T.vi"("what points"=w214, "temperature points"=w202) -> ("best fit parameters"=w190:dbl[], "what points out"=w204:dbl[], "residue"=→"residue left":dbl)  [unwired: 5 in, 2 out]
            "best fit parameters left" <- w190
            n125 = call "fit function -1 over T.vi"("X"=w189, "a"=w197) -> ("f(X,a)"=w184:dbl[])  [unwired: 2 in, 2 out]
            n126 = call "fit function -1 over T.vi"("X"=w185, "a"=w190) -> ("f(X,a)"=w183:dbl[])  [unwired: 2 in, 2 out]
            n127 = Subtract(x=w184, y=w183) -> (x-y=→"x-y":dbl[])
            n128 = Bundle(w209, "what points out"=w205) -> (w206:cluster{dbl[], "what points out":dbl[]})  [unwired: 1 in]
            n129 = Bundle(w208, "what points out"=w204) -> (w207:cluster{dbl[], "what points out":dbl[]})  [unwired: 1 in]
            n130 = Build Array(w210, w207, w206) -> (→"Plot:   what vs temp 2":T13)
          }
          frame "read rusout file" {
            n131 = Build Path(base path=w241, name or relative path="rusout.dat") -> (appended path=w239:path)
            n132 = call "link -- read rusout file - tetragonal.vi"("rus out file path"=w239, "buttons"=w237) -> ("Cluster out"=→"rusout file":T5, "all peaks exp"=→"all peaks exp":i32[], "array of coefficients"=w235:dbl[][], "Array of dL"=→"Array of dL":dbl[][])  [unwired: 4 in, 2 out]
            n133 = Array Size(array=w235) -> (size(s)=→"size(s)":i32[])
            n134 = local write "array of coefficients"(w235) -> ()
          }
          frame "calc el consts" {
            n135 = call-poly <vilib>:"Array To Matrix.vi"("Real 2D Array"=w253) -> ("Real Matrix"=w252:T14)
            n136 = Transpose Matrix(1:w252) -> (0:w245:T14)
            n137 = Matrix Size(0:w245) -> (1:→"number of rows 2":i32, 2:→"number of columns 2":i32)
            n138 = for {
              tunnel: w257 -> [w263] mode=indexing
              tunnel: [w262] -> w256 mode=indexing
              tunnel: [w261] -> w250
              n139 = Unbundle(w263) -> ("temperature points OUT"=w261:dbl[], w262:dbl[])
            }
            n140 = call-poly <vilib>:"Array To Matrix.vi"("Real 2D Array"=w256) -> ("Real Matrix"=w251:T14)
            n141 = call-poly <vilib>:"A x B.vi"("B"=w251, "A"=w245) -> ("A x B"=w242:T14)  [unwired: 1 out]
            n142 = Matrix Size(0:w242) -> (1:→"number of rows 3":i32, 2:→"number of columns 3":i32)
            n143 = call-poly <vilib>:"Matrix To Array.vi"("Real Matrix"=w242) -> ("Real 2D Array"=w249:dbl[][])
            n144 = Matrix Size(0:w251) -> (1:→"number of rows":i32, 2:→"number of columns":i32)
            n145 = for {
              tunnel: w250 -> [w260]
              tunnel: w249 -> [w259] mode=indexing
              tunnel: [w258] -> w248 mode=indexing
              n146 = Bundle("temperature points OUT"=w260, "Real 2D Array"=w259) -> (w258:T15)  [unwired: 1 in]
            }
            "Plot:   elastic vs temp" <- w248
          }
        }
      }
      event "temperature mapping": Value Change {
        (unwired) u8 0 ("X Scale.Mapping Mode")
        n147 = event-data() -> ()  [unwired: 1 in, 2 out]
        n148 = control-ref of="Plot:   what vs temp (all points)"() -> (w268:refnum<vi>)
        n149 = property on="Property Node" class="XYGraph (strict)"(reference=w268) -> (reference out=w265:refnum<vi>, "XScale.Mapping Mode"=w267:u8)  [unwired: 1 in, 1 out]
        n150 = Increment(x=w267) -> (x+1=w269:u8)
        n151 = Quotient & Remainder(x=w269, y=u8 2 ("X Scale.Mapping Mode")) -> (x-y*floor(x/y)=w264:u8)  [unwired: 1 out]
        n152 = property on="Property Node" class="XYGraph (strict)"(reference=w265, "XScale.Mapping Mode"=w264) -> ()  [unwired: 1 in, 2 out]
      }
      event "dump optimal vectors": Value Change {
        n153 = event-data() -> ()  [unwired: 1 in, 2 out]
        n154 = Generate User Event(user event=w271, event data cluster="dump optimal vectors" ("event data")) -> ()  [unwired: 2 in, 2 out]
      }
      event "what query": Value Change {
        n155 = event-data() -> ("OldVal"=w277:T2[], "NewVal"=w278:T2[])  [unwired: 1 in]
        n156 = flat-sequence {
          tunnel: w278 -> [w285]
          tunnel: w277 -> [w281]
          tunnel: w276 -> [w280]
          tunnel: [w280] -> w275
          tunnel: w274 -> [w279]
          tunnel: w275 -> [w286]
          frame #0 {
            n157 = call "query logic.vi"("type"=enum16{"selector", "send"}."selector", "OldVal"=w281, "NewVal"=w285) -> ("Numeric"=w284:i32, "NewVal  OUT"=w283:T2[])  [unwired: 6 in, 1 out]
            n158 = local write "what query"(w283) -> ()
            n159 = property class="Enum (strict)"(reference=w279, "Value"=w284) -> ()  [unwired: 1 in, 2 out]
          }
          frame #1 {
            n160 = Generate User Event(user event=w286, event data cluster="recalculate" ("event data")) -> ()  [unwired: 2 in, 2 out]
          }
        }
      }
      event "Plot:   what vs temp": Cursor Release; "gap": Value Change {
        w289 = "critical"  # action
        n161 = event-data() -> ()  [unwired: 1 in, 1 out]
        n162 = Generate User Event(user event=w288, event data cluster=w289) -> ()  [unwired: 2 in, 2 out]
      }
      event "read/write buttons": Value Change {
        n163 = event-data() -> ("OldVal"=w290:T2[], "NewVal"=w294:T2[])  [unwired: 1 in, 4 out]
        n164 = call "query logic.vi"("type"=enum16{"selector", "send"}."send", "OldVal"=w290, "NewVal"=w294) -> ("selector"=w292:string, "NewVal  OUT"=w293:T2[])  [unwired: 6 in, 1 out]
        n165 = case shown="\"write buttons\"" w292 {
          tunnel: [enum16{"read", "none", "write"}."none" ("what") enum16{"read", "none", "write"}."write" ("what") enum16{"read", "none", "write"}."read" ("what")] -> w295
          frame "False", Default {
          }
          frame "write buttons" {
          }
          frame "read buttons" {
          }
        }
        n166 = call "rpr -- read write buttons.vi"("what"=w295, "appended array"=w297, "peaks"=w298, "9w folder path"=w296) -> ()  [unwired: 8 in]
        n167 = local write "read/write buttons"(w293) -> ()
      }
      event "temperature mapping": Value Change {
        n168 = event-data() -> ("OldVal"=w304:T2[], "NewVal"=w303:T2[])  [unwired: 1 in, 3 out]
        n169 = call "query logic.vi"("type"=enum16{"selector", "send"}."selector", "OldVal"=w304, "NewVal"=w303) -> ("selector"=w302:string)  [unwired: 6 in, 2 out]
        n170 = case shown="\"linear\"" w302 {
          frame "False", Default {
          }
          frame "linear" {
            w306 = u8 1 ("X Scale.Mapping Mode")
            n171 = property on="Plot:   what vs temp (all points)" class="XYGraph (strict)"("XScale.Mapping Mode"=w306) -> ()  [unwired: 2 in, 2 out]
            n172 = property on="Plot:   what vs temp" class="XYGraph (strict)"("XScale.Mapping Mode"=w306) -> ()  [unwired: 2 in, 2 out]
          }
          frame "logarithmic" {
            w307 = u8 0 ("X Scale.Mapping Mode")
            n173 = property on="Plot:   what vs temp (all points)" class="XYGraph (strict)"("XScale.Mapping Mode"=w307) -> ()  [unwired: 2 in, 2 out]
            n174 = property on="Plot:   what vs temp" class="XYGraph (strict)"("XScale.Mapping Mode"=w307) -> ()  [unwired: 2 in, 2 out]
          }
        }
      }
      event "active": Value Change {
        n175 = event-data() -> ("OldVal"=w311:bool[], "NewVal"=w310:bool[])  [unwired: 1 in]
        n176 = flat-sequence {
          tunnel: w311 -> [w318]
          tunnel: w310 -> [w317]
          tunnel: w308 -> [w312]
          tunnel: w309 -> [w329]
          frame #0 {
            n177 = for {
              tunnel: w318 -> [w320] mode=indexing
              tunnel: w317 -> [w319] mode=indexing
              tunnel: [w325] -> w315 mode=indexing
              shift-right: [w324] -> w314
              shift-left: 0 -> [w322]
              i -> [w323]
              n178 = Not(x=w320) -> (.not. x?=w321:bool)
              n179 = And(x=w321, y=w319) -> (x .and. y?=w325:bool)
              n180 = case shown="False" w325 {
                tunnel: [w326 w327] -> w324
                tunnel: w323 -> [_ w327]
                tunnel: w322 -> [w326 _]
                frame False {
                }
                frame True {
                }
              }
            }
            "Numeric" <- w314
            n181 = local write "active"(w315) -> ()
            n182 = Index Array(array=w312, index=w314) -> (element=w313:refnum<vi>)
            n183 = local write "active buttons ref"(w313) -> ()
          }
          frame #1 {
            w328 = "recalculate"  # action
            n184 = Generate User Event(user event=w329, event data cluster=w328) -> ()  [unwired: 2 in, 2 out]
          }
        }
      }
      event "Plot:   what vs temp (all points)": Cursor Move {
        # "window  cursor bracket"
        n185 = event-data() -> ("CursIdx"=w332:i32)  [unwired: 1 in, 4 out]
        n186 = control-ref of="Plot:   what vs temp (all points)"() -> ()  [unwired: 1 out]
        n187 = call "cursor window logic.vi"("CursIdx"=w332, "cursor window action"=cursor_window_action."cursor moves", "cursor bracket in"=w331) -> ()  [unwired: 7 in, 2 out]
      }
      event "Plot:   what vs temp": Cursor Move {
        # "window  cursor bracket"
        n188 = event-data() -> ("CursIdx"=w336:i32)  [unwired: 1 in]
        n189 = control-ref of="Plot:   what vs temp (all points)"() -> ()  [unwired: 1 out]
        n190 = call "cursor window logic.vi"("CursIdx"=w336, "cursor window action"=cursor_window_action."cursor moves", "cursor bracket in"=w334) -> ("cursor window out"=w333:T4)  [unwired: 7 in, 1 out]
        n191 = Unbundle By Name(w333) -> ()  [unwired: 1 out]
      }
      event "Plot:   what vs temp (all points)": Mouse Move {
        w342 = 0
        n192 = event-data() -> ("Coords"=w356:T16)  [unwired: 1 in]
        n193 = control-ref of="Plot:   what vs temp (all points)"() -> (w355:refnum<vi>)
        n194 = Initialize Array(w342, w342) -> (w341:i32[])
        n195 = invoke class="XYGraph (strict)" method="Map Coords To XY"(reference=w355, "Coords"=w356) -> ("XY"=w353:cluster{"X":dbl, "Y":dbl})  [unwired: 5 in, 6 out]
        n196 = for {
          tunnel: w343 -> [w357] mode=indexing
          shift-right: [w358] -> _
          shift-left: w341 -> [w359]
          i -> [w360]
          n197 = case shown="False" w357 {
            tunnel: w360 -> [_ w364]
            tunnel: w359 -> [w361 w363]
            tunnel: [w361 w362] -> w358
            frame False {
            }
            frame True {
              n198 = Build Array (concatenate)(w363, w364) -> (w362:i32[])
            }
          }
        }
        n199 = local read "common temperature points"() -> (w352:dbl[])
        n200 = local read "common  freq points"() -> (w351:dbl[][])
        n201 = Unbundle By Name(w353) -> ("X"=w354:dbl, "Y"=w348:dbl)
        n202 = Threshold 1D Array(2:w354, 3:w352) -> (0:w350:dbl)  [unwired: 1 in]
        n203 = Index Array(array=w351, index (col)=w350) -> (element=w347:dbl[])  [unwired: 1 in]
        n204 = local read "Array of dL"() -> (w340:dbl[][])
        n205 = local read "peaks -- used"() -> (w349:i32[])
        n206 = local read "rusout file"() -> (w344:T5)
        n207 = Subtract(x=w347, y=w348) -> (x-y=w346:dbl[])
        n208 = Unbundle By Name(w344) -> ()  [unwired: 6 out]
        n209 = Square(x=w346) -> (x^2=w345:dbl[])
        n210 = Array Max & Min(array=w345) -> (min index (indices)=w337:i32)  [unwired: 3 out]
        n211 = Index Array(array=w349, index=w337) -> (element=→"element":i32)
        n212 = Index Array(array=w340, index (row)=w337) -> (element=→"subarray":dbl[])  [unwired: 1 in]
      }
      event "show plot pallettes": Value Change {
        n213 = event-data() -> ("NewVal"=w367:bool)  [unwired: 1 in, 1 out]
        n214 = property on="Plot:   optimal subspace" class="XYGraph (strict)"("ScaleLegendVis"=w367, "Palette Visible"=w367, "Legend Visible"=w367) -> ()  [unwired: 2 in, 2 out]
        n215 = property on="Plot:   elastic vs temp" class="XYGraph (strict)"("ScaleLegendVis"=w367, "Palette Visible"=w367, "Legend Visible"=w367) -> ()  [unwired: 2 in, 2 out]
        n216 = property on="Plot:   what vs temp (all points)" class="XYGraph (strict)"("ScaleLegendVis"=w367, "Palette Visible"=w367, "Legend Visible"=w367) -> ()  [unwired: 2 in, 2 out]
        n217 = property on="Plot:   what vs temp" class="XYGraph (strict)"("ScaleLegendVis"=w367, "Palette Visible"=w367, "Legend Visible"=w367) -> ()  [unwired: 2 in, 2 out]
        n218 = call "cursor window logic.vi"("cursor window action"=cursor_window_action."check", "cursor bracket in"=w366) -> ()  [unwired: 8 in, 2 out]
      }
      event "misc controls": Value Change {
        n219 = event-data() -> ("OldVal"=w369:T2[], "NewVal"=w372:T2[])  [unwired: 1 in, 2 out]
        n220 = call "query logic.vi"("type"=enum16{"selector", "send"}."send", "OldVal"=w369, "NewVal"=w372) -> ("selector"=w370:string, "NewVal  OUT"=w371:T2[])  [unwired: 6 in, 1 out]
        n221 = local write "misc controls"(w371) -> ()
        n222 = Generate User Event(user event=w373, event data cluster=w370) -> ()  [unwired: 2 in, 2 out]
      }
      event "buttons 2", "buttons 3", "buttons 4", "buttons 1": Value Change {
        w374 = "recalculate"  # action
        n223 = event-data() -> ()  [unwired: 1 in, 5 out]
        n224 = Generate User Event(user event=w375, event data cluster=w374) -> ()  [unwired: 2 in, 2 out]
      }
      event "Plot:   what vs temp (all points)": Cursor Release {
        w377 = "recalculate"  # action
        n225 = event-data() -> ()  [unwired: 1 in, 8 out]
        n226 = Generate User Event(user event=w376, event data cluster=w377) -> ()  [unwired: 2 in, 2 out]
      }
      event Timeout {
        n227 = event-data() -> ()  [unwired: 1 in, 2 out]
      }
    }
    n228 = Wait (ms)(milliseconds to wait=w71) -> ()  [unwired: 1 out]
  }
